vi "Main.vi"() -> ()   [LabVIEW 2024]
uses:
  SubVIs/Typdefinitionen/Zustand.ctl
  SubVIs/Typdefinitionen/Registerkartenelement.ctl
  SubVIs/Typdefinitionen/Cluster_SPS_IN.ctl
  SubVIs/Typdefinitionen/Befehl_Lichtgitter.ctl
  SubVIs/Typdefinitionen/Cluster_out_Lichtgitter.ctl
  SubVIs/Typdefinitionen/Statistik.ctl
  SubVIs/Typdefinitionen/Cluster_SPS_OUT.ctl
  <vilib>/vision/Image Controls.llb/IMAQ Image.ctl
  SubVIs/Sonstige/Globale Variablen.vi
  <vilib>/vision/driver/NI_Vision_Acquisition_Software.lvlib
panel:
  out "error out":errorcluster
  in  "Registerkarte":T1
  in  "Start Kamera Unten":bool
  in  "Start Position":bool
  in  "Start Lichtgitter":bool
  in  "Zoom zurücksetzen":bool
  in  "Registerkarte Bilder":enum32{"Prüfungen", "Rohbilder"}(tab)
  out "Nachprüfung von Unten":T2(plugin-control)
  out "Ermittlung Kontaktposition":T2(plugin-control)
  out "Rohbild ISO":T2(plugin-control)
  out "Rohbild Referenzmarken":T2(plugin-control)
  out "Zeit Position ermitteln (ms)":u32
  out "Zeit Lichtgitter (ms)":u32
  out "Zeit Kamera Unten (ms)":u32
  in  "Größe Kontaktsuchfeld":sgl=70.0
  out "Artikelnummer & Fertigungsauftrag":T3={"Artikelnummer"="Test", "Fertigungsauftrag"="Test"}
  out "Messdaten":T4 {"Durchmesser Kontakt" format="%#.3f"; "Durchmesser Loch" format="%#.3f"; "Winkel Kontakt" format="%#.0f"; "Offset"."x" format="%#.3f"; "Offset"."y" format="%#.3g"; "Position Kontakt"."x" format="%#.3f"; "Position Kontakt"."y" format="%#.3f"}
  in  "Offline":T5={"Start Gesamtablauf"=FALSE, "Teile-Nummer"=0, "Teile-Datum"=0, "Kontaktnummer"=1} {"Kontaktnummer" min=1 max=40 step=1; "Teile-Datum" items=["09.12.24"]; "Teile-Nummer" max=0 step=1}
  out "Statistik Anlage":T6
  out "Statistik Artikel":T6
  out "Statistik Auftrag":T6
  out "SPS IN":T7
  out "SPS OUT":T8
  in  "Bildspeicherung Offline":bool
  in  "Cluster beobachten":bool
  in  "Lichtgitter manuell ansteuern":bool
  in  "Befehl:":T9
  out "Ergebnisse:":T10
  in  "ID Messverstärker":u32=1 min=1 max=2
  in  "Artikelnummer Offline":string="Test"
  in  "i. O. Bilder speichern":bool
  in  "SubVI öffnen":bool
  in  "Livebild":bool
  out "Zustand":T11=enum."Bild Unten speichern"
  out "Programmversion":string
  in  "ACK":bool
  out "Beschreibung:":string
  in  "Fehlercode:":string
  out "Fehler Beenden":errorcluster
  in  "Flüssiglinse neu verbinden":bool
  out "Fehler Flüssiglinse":errorcluster
  in  "Lichtgitter neu verbinden":bool
  in  "SPS neu verbinden":bool
  in  "Kamera Oben neu verbinden":bool
  in  "Kamera Unten neu verbinden":bool
  out "Fehler Lichtgitter":errorcluster
  out "Fehler SPS":errorcluster
  out "Fehler Kamera Unten":errorcluster
  out "Fehler Kamera Oben":errorcluster
  out "Fehler init allgemein":errorcluster
  out "Fehler Nebenschleife":errorcluster
  out "Fehler Main":errorcluster
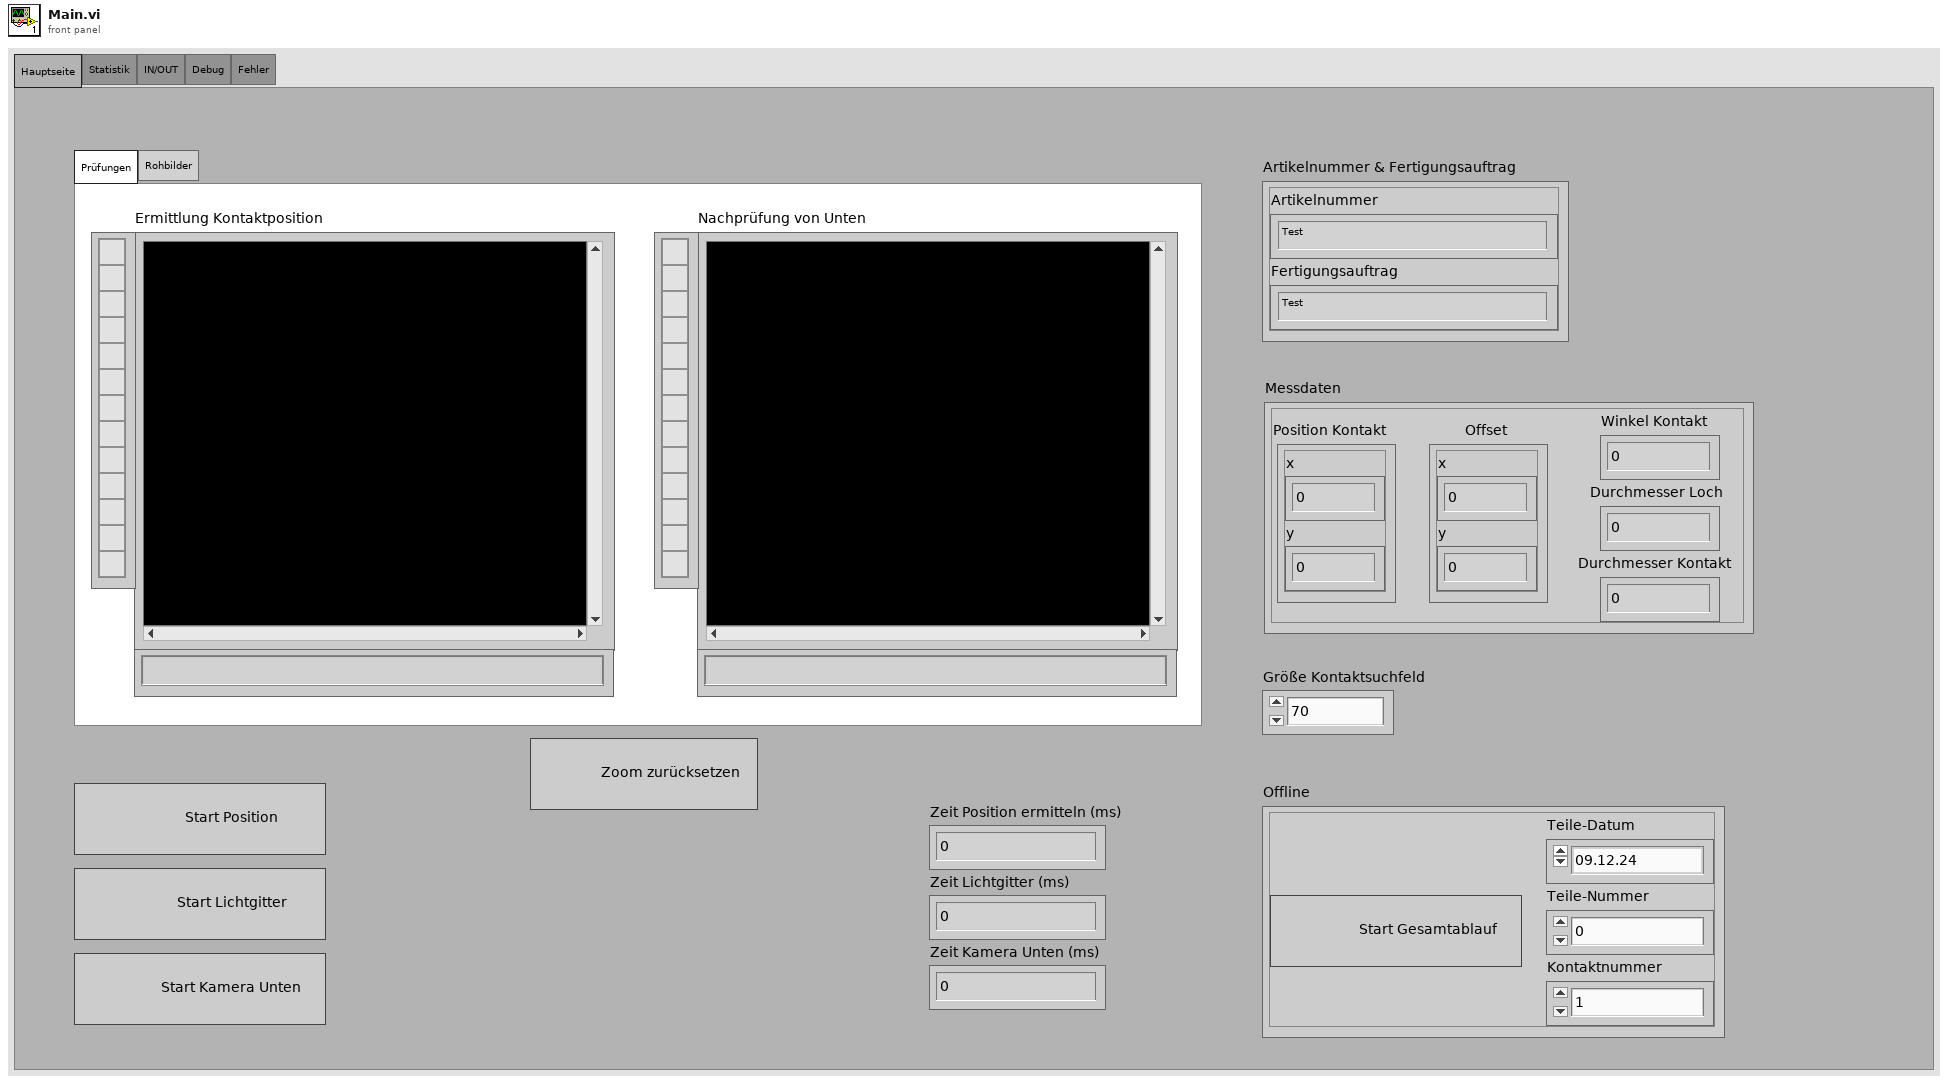
[diagram p1: front panel]
types:
  T1 = typedef "Registerkartenelement.ctl" = enum32{"Hauptseite", "Statistik", "IN/OUT", "Debug", "Fehler"}
  T2 = typedef "IMAQ Image.ctl" = refnum<image>
  T3 = cluster{"Artikelnummer":string, "Fertigungsauftrag":string}
  T4 = cluster{"Position Kontakt":cluster{"x":dbl, "y":dbl}, "Offset":cluster{"x":dbl, "y":dbl}, "Winkel Kontakt":dbl, "Durchmesser Loch":dbl, "Durchmesser Kontakt":dbl}
  T5 = cluster{"Start Gesamtablauf":bool, "Teile-Nummer":u32, "Teile-Datum":u16, "Kontaktnummer":u32}
  T6 = typedef "Statistik.ctl" = cluster{"Bestückte ISO":u32, "Verbaute Kontakte":u32, "ISO n.i.O.":u32, "Nachkontrolle Unten n.i.O":u32, "Position nicht gefunden":u32}
  T7 = typedef "Cluster_SPS_IN.ctl" = cluster{"Artikelnummer":string, "Fertigungsauftrag":string, "Start Position ermitteln":bool, "Start Kontaktvermessung Lichtgitter":bool, "Start Nachkontrolle":bool, "ACK SPS":bool}
  T8 = typedef "Cluster_SPS_OUT.ctl" = cluster{"Koordinaten ermittelt":bool, "Nachkontrolle Kamera Unten fertig":bool, "Vermessung Lichtgitter fertig":bool, "Position x":dbl, "Position y":dbl, "Winkel Kontakt":dbl, "Offset x":dbl, "Offset y":dbl, "Referenzen nicht gefunden":bool, "Kontaktposition nicht gefunden":bool, "Kontakt nicht in Lichtgitter":bool, "Kontakt zu klein":bool, "Kontakt zu groß":bool, "Kamera Unten n.i.O.":bool}
  T9 = typedef "Befehl_Lichtgitter.ctl" = enum16{"Anzahl Messverstärker ermitteln", "Aktuellen Messwert von einem Messverstärker lesen", "Aktuellen Messwerte von allen Messverstärkern lesen", "Anzahl Kanten von einem Messverstärker ermitteln", "Alle Kanten von allen Messverstärkern lesen"}
  T10 = typedef "Cluster_out_Lichtgitter.ctl" = cluster{"Anzahl Messverstärker":i32, "Messwert in mm":dbl, "Alle Messwerte in mm":dbl[], "Anzahl Kanten":i32, "Messwerte out":dbl[][]}
  T11 = typedef "Zustand.ctl" = enum16{"Warten auf Event", "Artikeldaten laden", "Init Prüfung Oben", "Bildaufnahme Oben", "Auswertung Oben", "Bilder Oben speichern", "Init Vermessung Lichtgitter", "Messwertaufnahme Lichtgitter", "Auswertung Lichtgitter", "Init Prüfung Unten", "Bildaufnahme Unten", "Auswertung Unten", "Bild Unten speichern", "Update Statistik", "Fehler quittieren"}
  T12 = enum32{"invalid app kind", "Development System", "Run Time System", "Student Edition", "Embedded LabVIEW", "Evaluation", "Custom"}
  T13 = typedef "Cluster_Fehler_Initialisierung.ctl" = cluster{"Fehler init allgemein":errorcluster, "Fehler Kamera Oben init":errorcluster, "Fehler Flüssiglinse init":errorcluster, "Fehler Kamera Unten init":errorcluster, "Fehler SPS init":errorcluster, "Fehler Lichtgitter init":errorcluster}
  T14 = typedef "Cluster.ctl" = cluster{"Initialisierung":cluster{"Online?":bool, "Grundpfad":path, "Kamera Oben":T15, "IP-Adresse Flüssiglinse":string, "Flüssiglinse":refnum<k5>, "Kamera Unten":T15, "IP-Adresse SPS":string, "SPS-Verbindung":T16, "IP-Adresse Lichtgitter":string, "Lichtgitter":refnum<k5>, "Skalierungsfaktor":dbl, "Bilder Oben":T2[], "Bild Unten":T2, "Bild Ausschnitt Unten":T2}, "Einstellungen":cluster{"Gesamtablauf gestartet":bool, "i. O. Bilder speichern":bool, "Bildspeicherung Offline":bool, "Ausgewähltes Offline-Datum":string, "Ausgewähltes Offline-Teil":string, "Speicherpfad Bilder":path}, "Artikeldaten":cluster{"Artikelnummer":string, "Fertigungsauftrag":string, "Muster ISO":T2, "Belichtungszeit Referenzmarken":dbl, "Fokus Referenzmarken":dbl, "Belichtungszeit ISO":dbl, "Fokus ISO":dbl, "Belichtungszeit Unten":dbl, "Kontaktanzahl":u32, "Aktueller Kontakt":i16, "Kontaktposition":cluster{"x":sgl, "y":sgl}, "ISO-Muster nicht vorhanden":bool, "Winkel ISO":sgl, "Mittelpunkt ISO":cluster{"x":dbl, "y":dbl}}, "Werte Kamera Oben":cluster{"Koordinatensystem":T19, "Position Kontakt":cluster{"x":dbl, "y":dbl}, "Durchmesser Loch":dbl, "Winkel Kontakt":dbl, "Position Kontakt umgerechnet":cluster{"x":dbl, "y":dbl}}, "Werte Kamera Unten":cluster{"Prüfung Unten n. i. O.":bool}, "Werte Lichtgitter":cluster{"Messwerte Referenzmarken":dbl[][], "Mittelpunkt Referenzmarken":cluster{"x":dbl, "y":dbl}, "Messwerte Kontakt":dbl[][], "Offset":cluster{"x":dbl, "y":dbl}}, "Rückmeldungen":cluster{"Koordinaten ermittelt":bool, "Vermessung Lichtgitter fertig":bool, "Nachkontrolle Kamera Unten fertig":bool}, "Fehler":cluster{"Referenzen nicht gefunden":bool, "Kontakt nicht gefunden":bool, "Referenzen nicht in Lichtgitter":bool, "Kontakt zu groß":bool, "Kontakt zu klein":bool}, "Statistik":cluster{"Statistiken":T6[]}, "Timer":cluster{"Timer Start Position":u32, "Timer Start Lichtgitter":u32, "Timer Start Kamera Unten":u32}}
  T15 = typedef "IMAQdx.ctl" = refnum<k21>
  T16 = typedef "SP7.lvlib/S7 Connection.ctl" = cluster{"TCP Connection Ref":refnum<k5>, "IP address":string, "timeout ms":i32, "Connected?":bool, "PLC Type":T17, "Rack S7 400":u8, "Slot S7 400":u8, "PDU Size":u16, "connection semaphore":T18}
  T17 = typedef "SP7.lvlib/PLC Type.ctl" = enum16{"S7 200", "S7 300/400", "S7 1200", "S7 1500", "LOGO!8"}
  T18 = typedef "Semaphore RefNum" = refnum<k1>
  T19 = typedef "Koordinatensystem.ctl" = cluster{"Punkt x-Achse":cluster{"X":sgl, "Y":sgl}, "Ursprung":cluster{"X":sgl, "Y":sgl}, "Punkt y-Achse":cluster{"X":sgl, "Y":sgl}}
  T20 = cluster{"Referenzen nicht gefunden":bool, "Kontakt nicht gefunden":bool, "Kontakt nicht in Lichtgitter":bool, "Kontakt zu groß":bool, "Kontakt zu klein":bool}
  T21 = cluster{"Messwerte Referenzmarken":dbl[][], "Mittelpunkt Referenzmarken":cluster{"x":dbl, "y":dbl}, "Messwerte Kontakt":dbl[][], "Offset":cluster{"x":dbl, "y":dbl}}
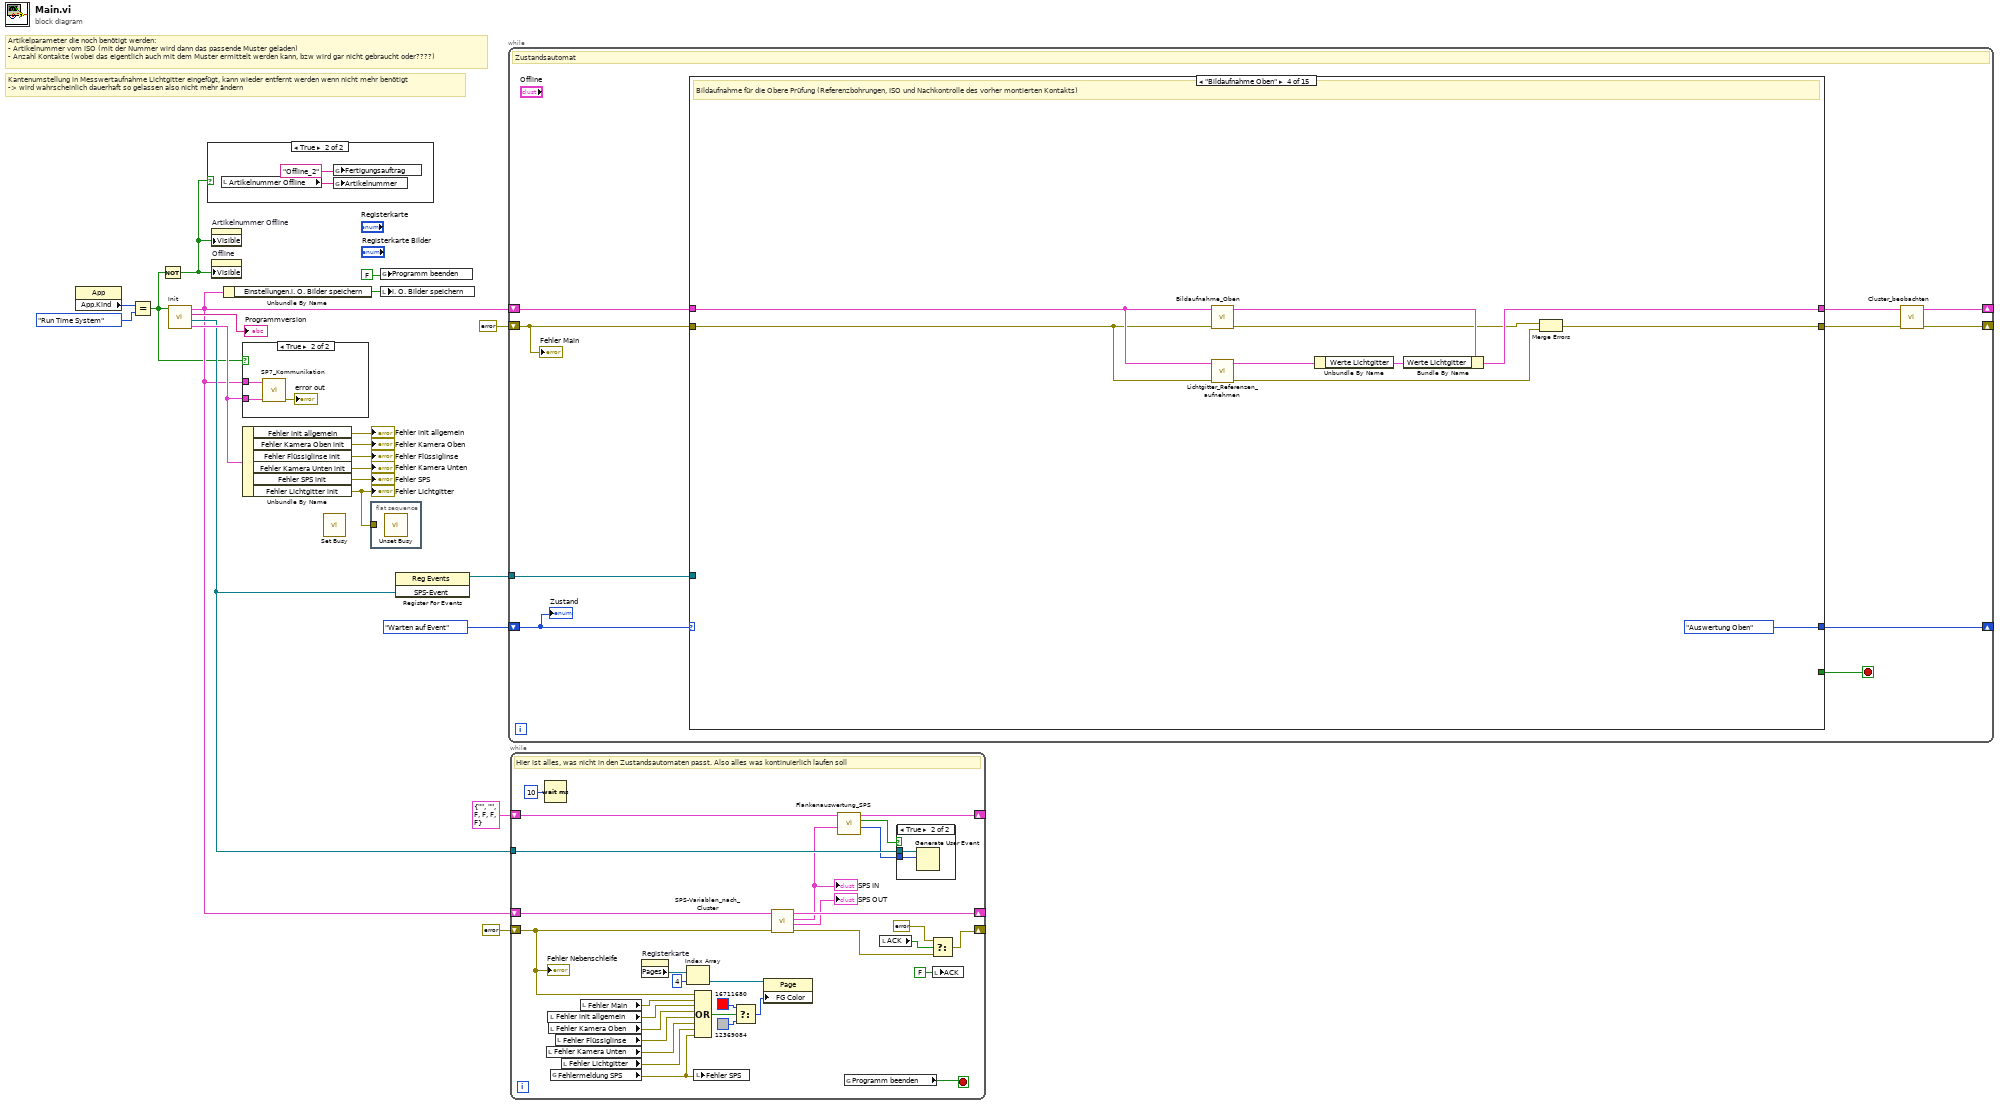
[diagram p0: block diagram]
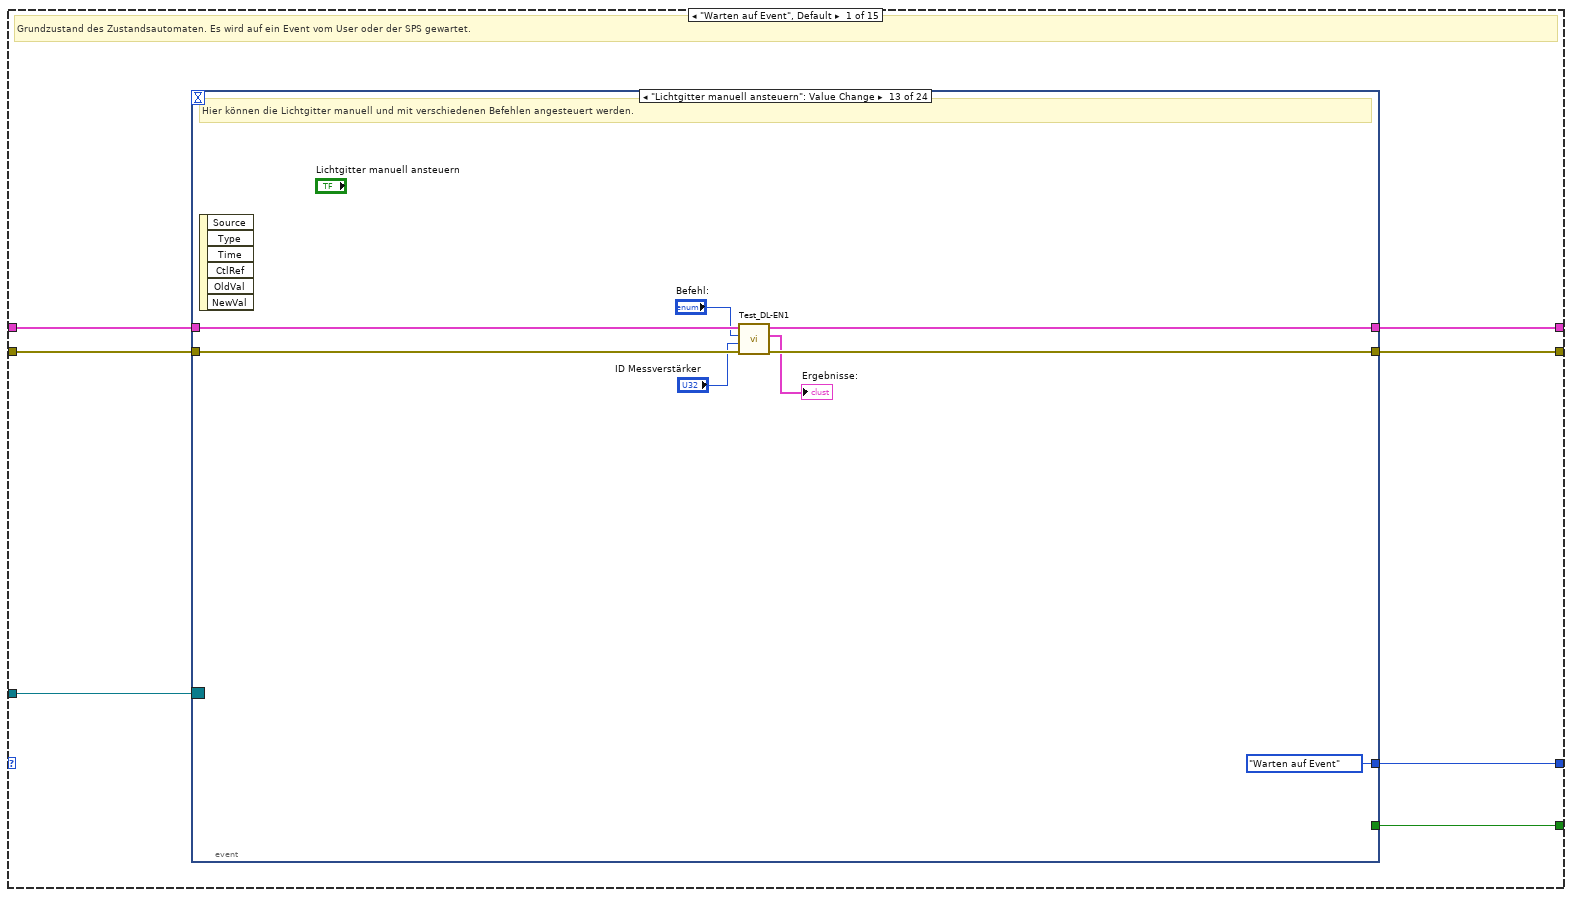
[diagram p2: hidden frame]
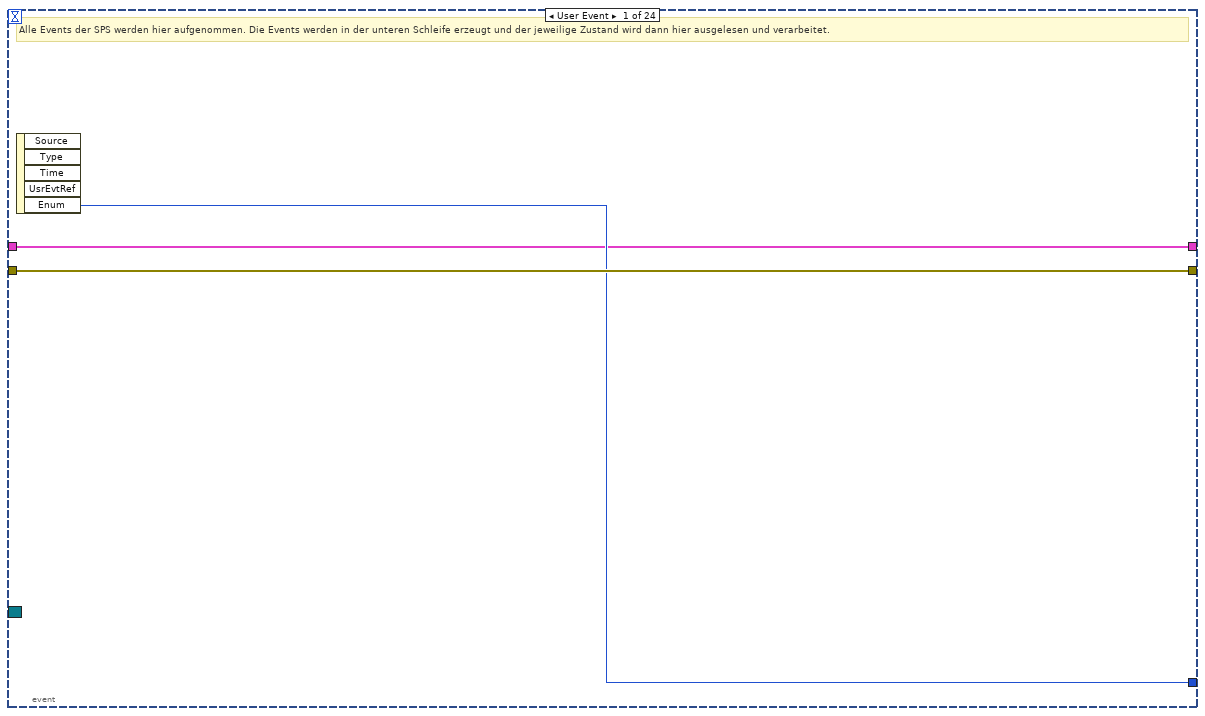
[diagram p3: hidden frame]
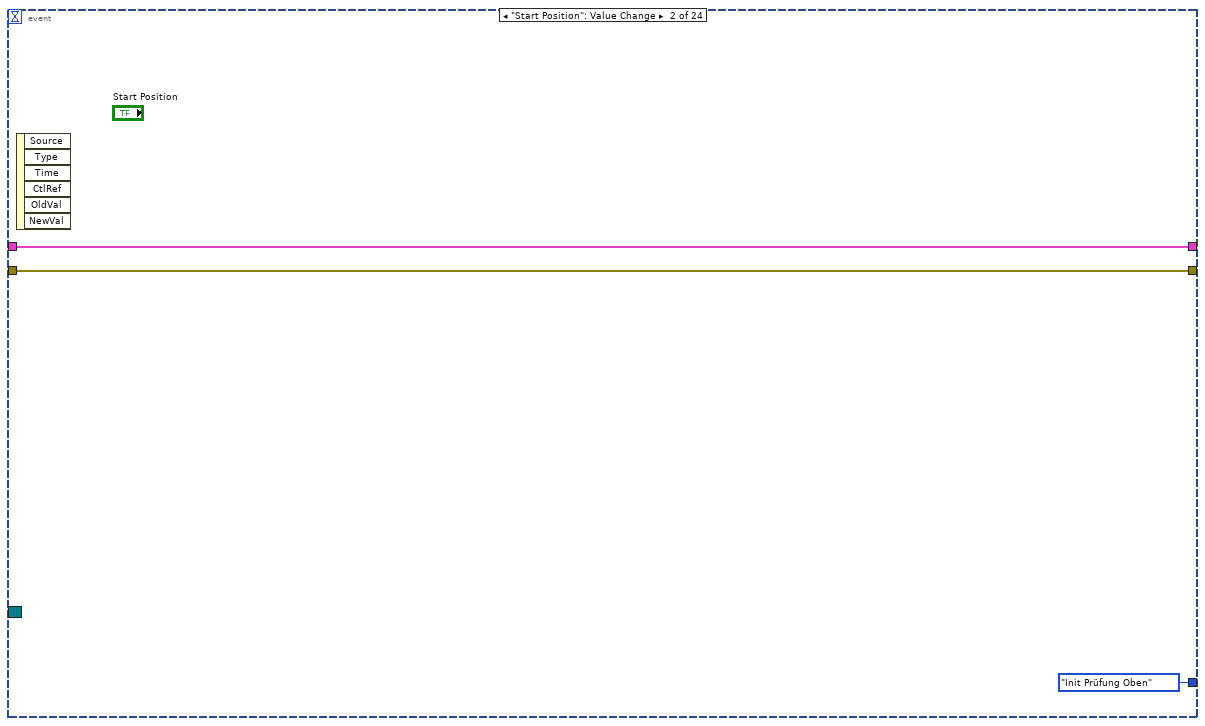
[diagram p4: hidden frame]
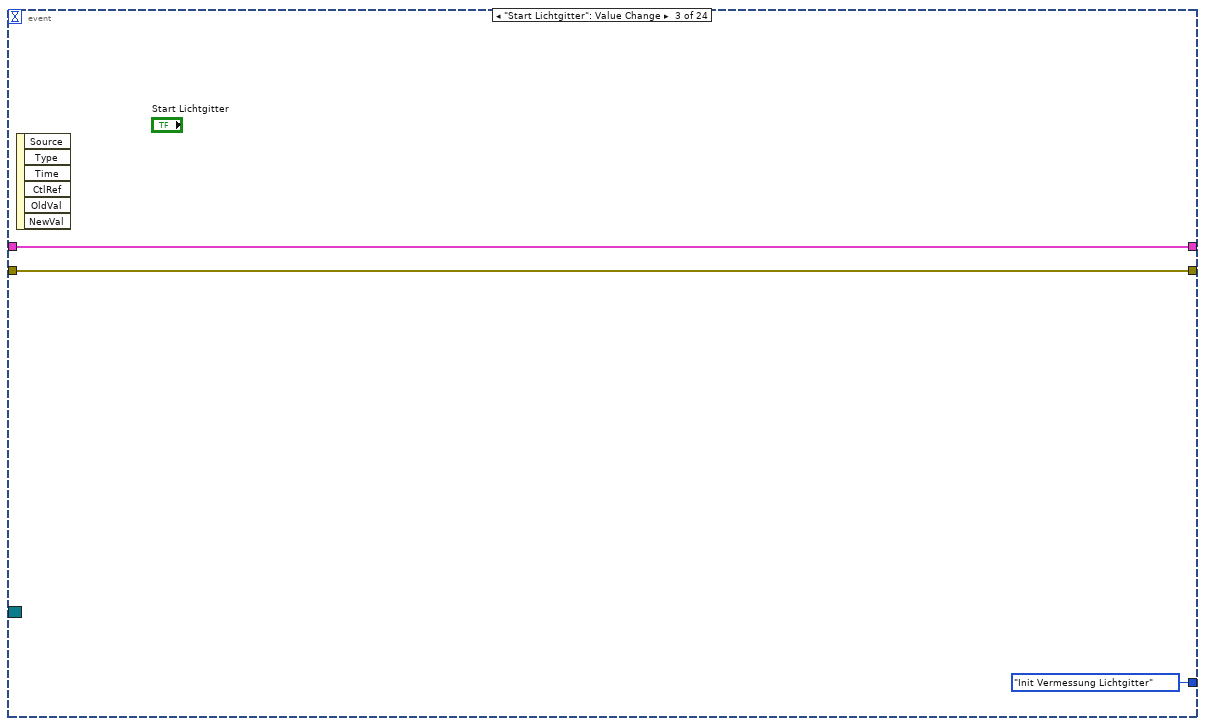
[diagram p5: hidden frame]
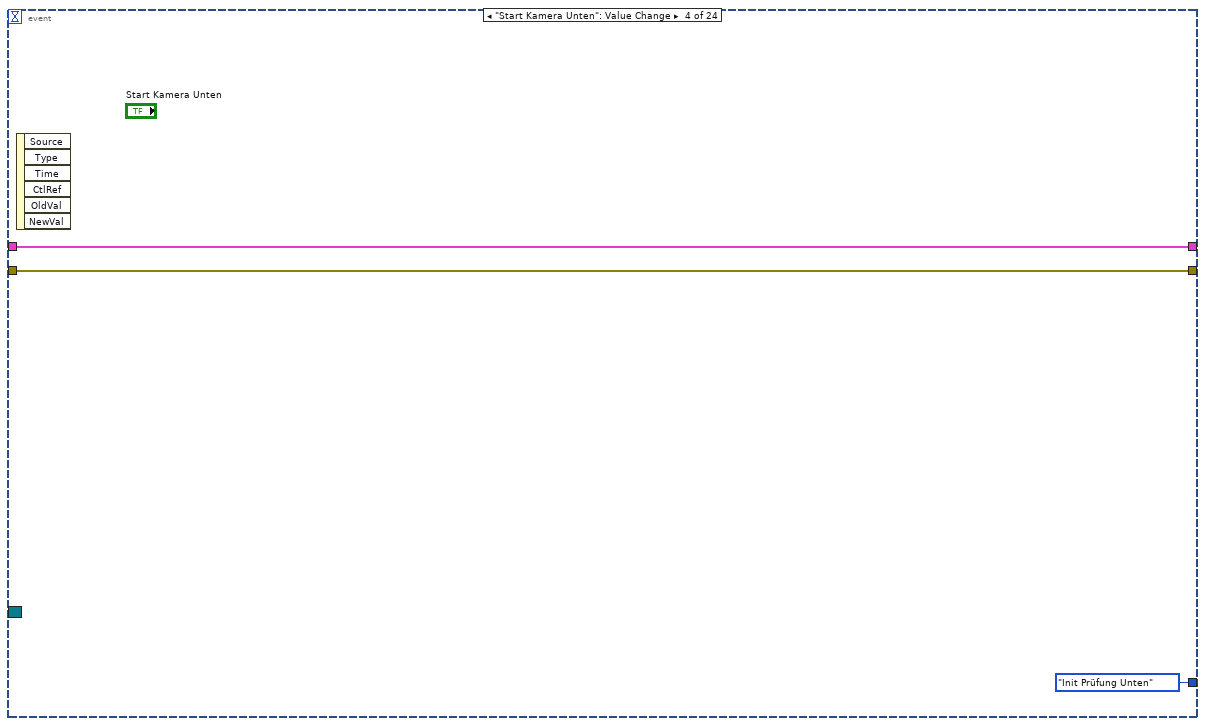
[diagram p6: hidden frame]
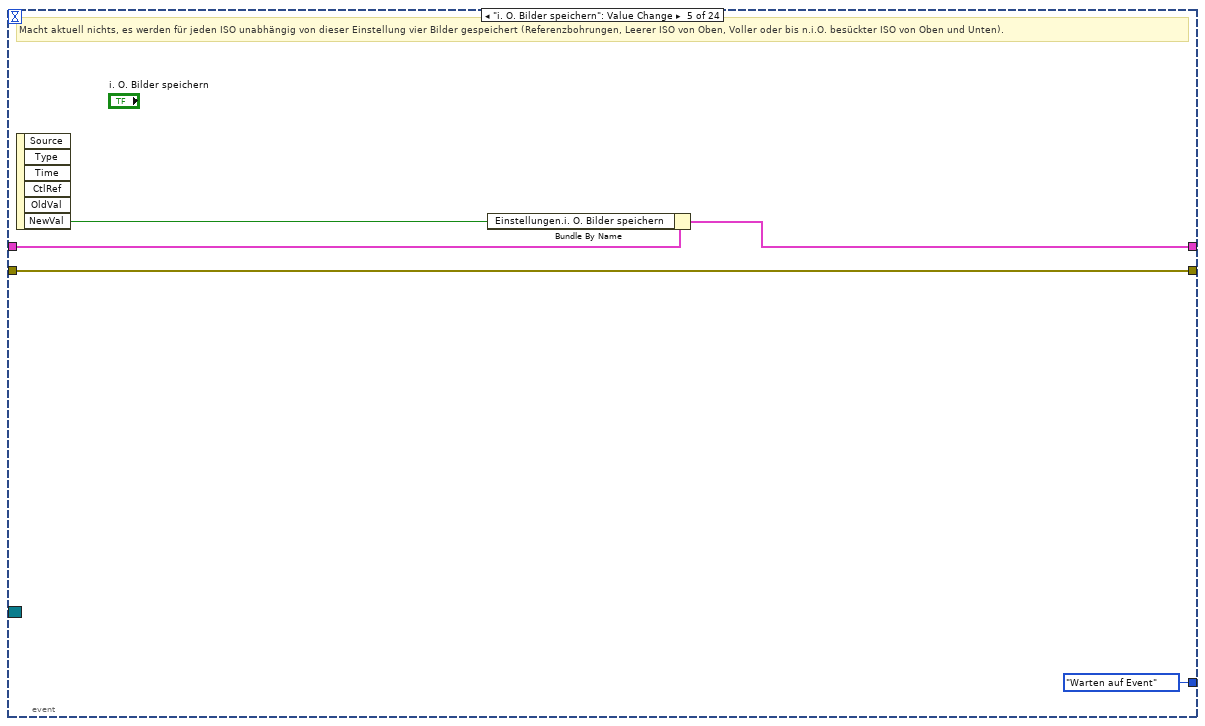
[diagram p7: hidden frame]
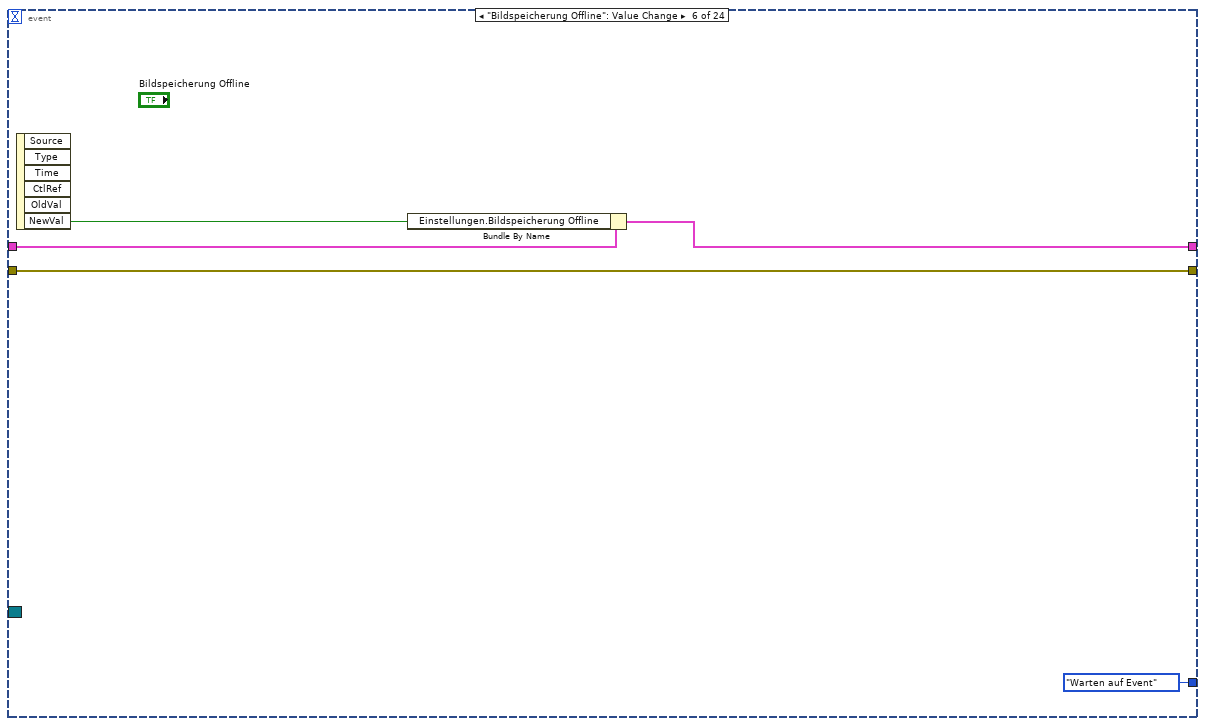
[diagram p8: hidden frame]
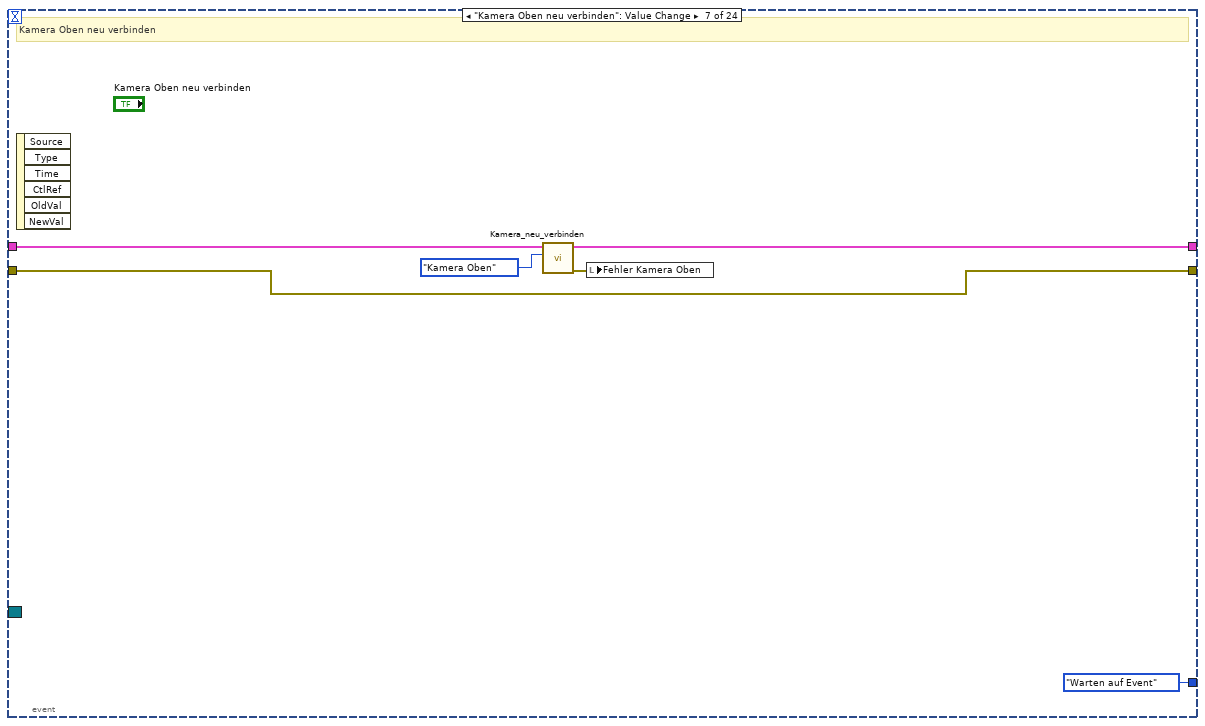
[diagram p9: hidden frame]
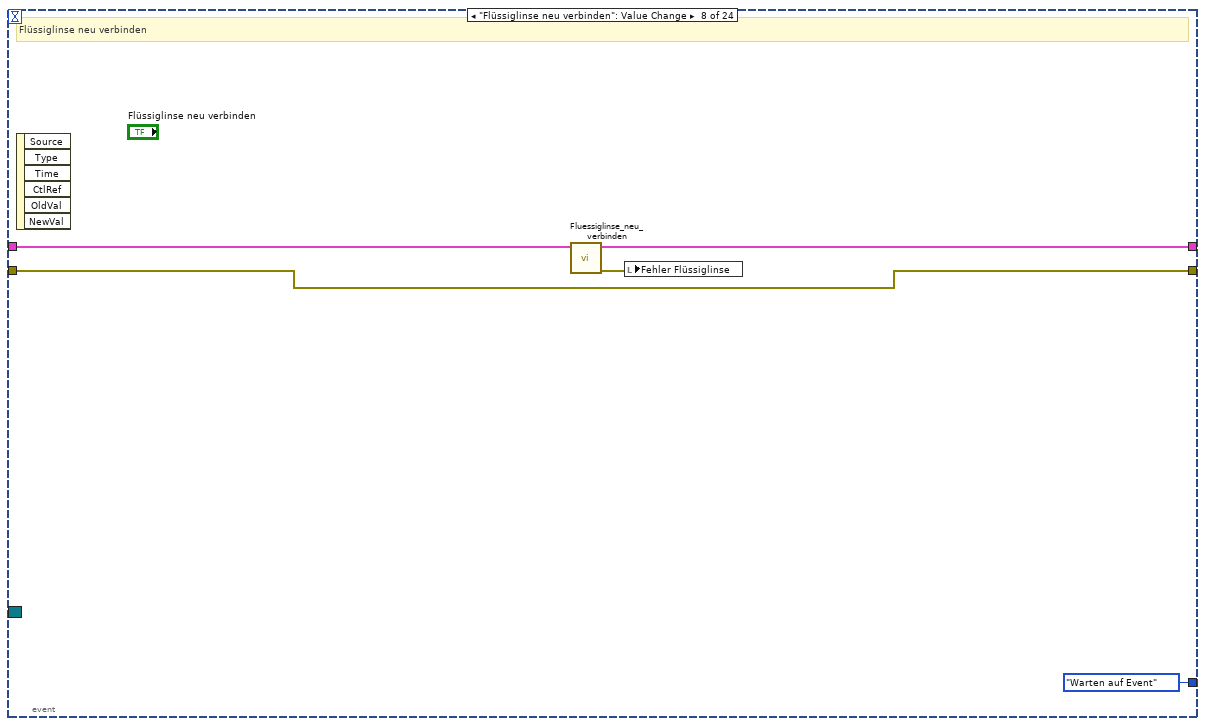
[diagram p10: hidden frame]
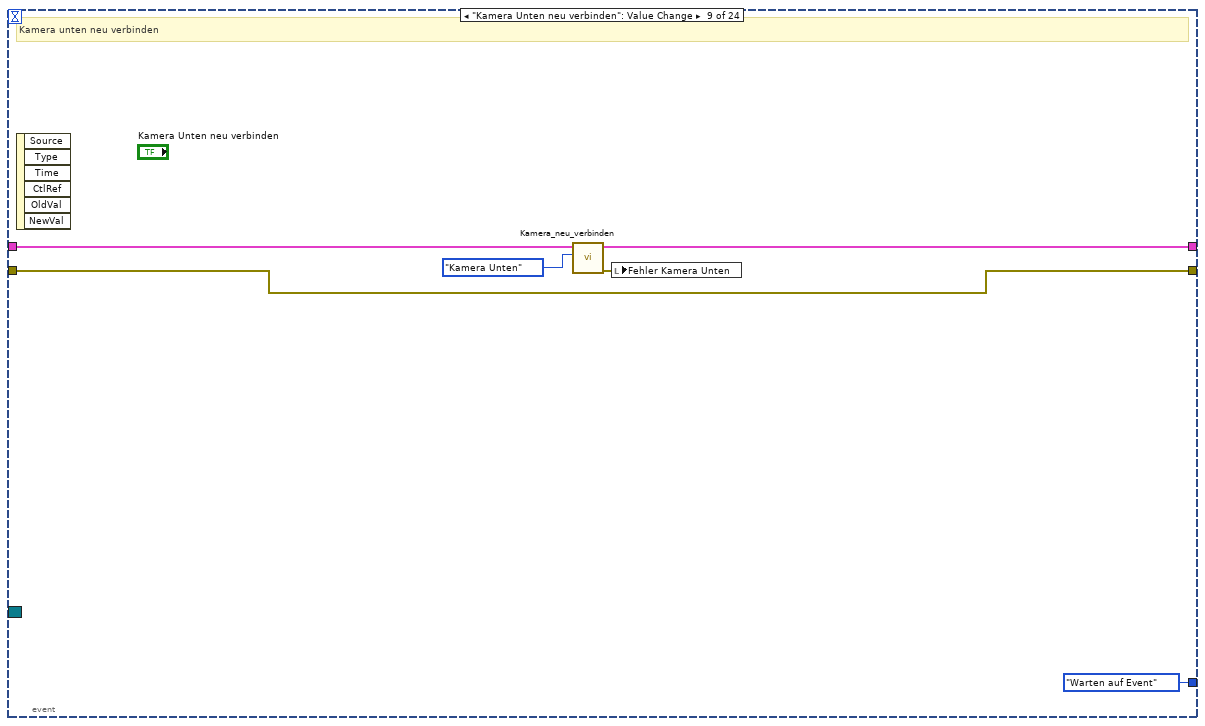
[diagram p11: hidden frame]
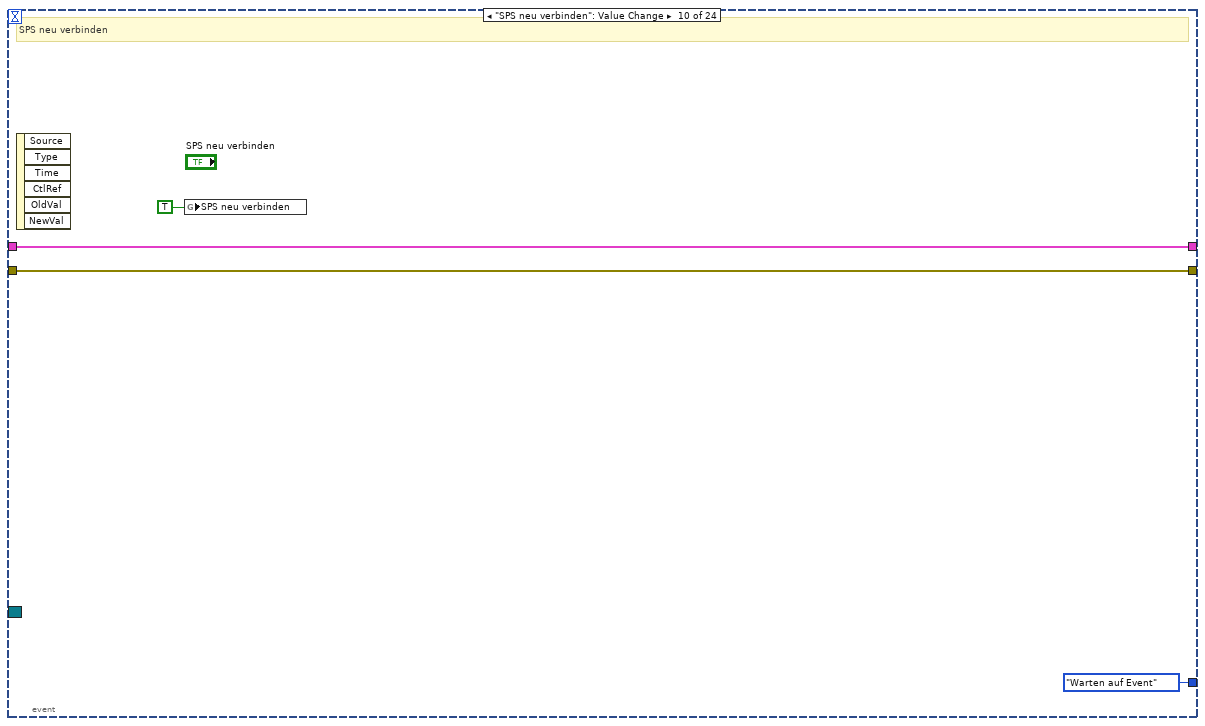
[diagram p12: hidden frame]
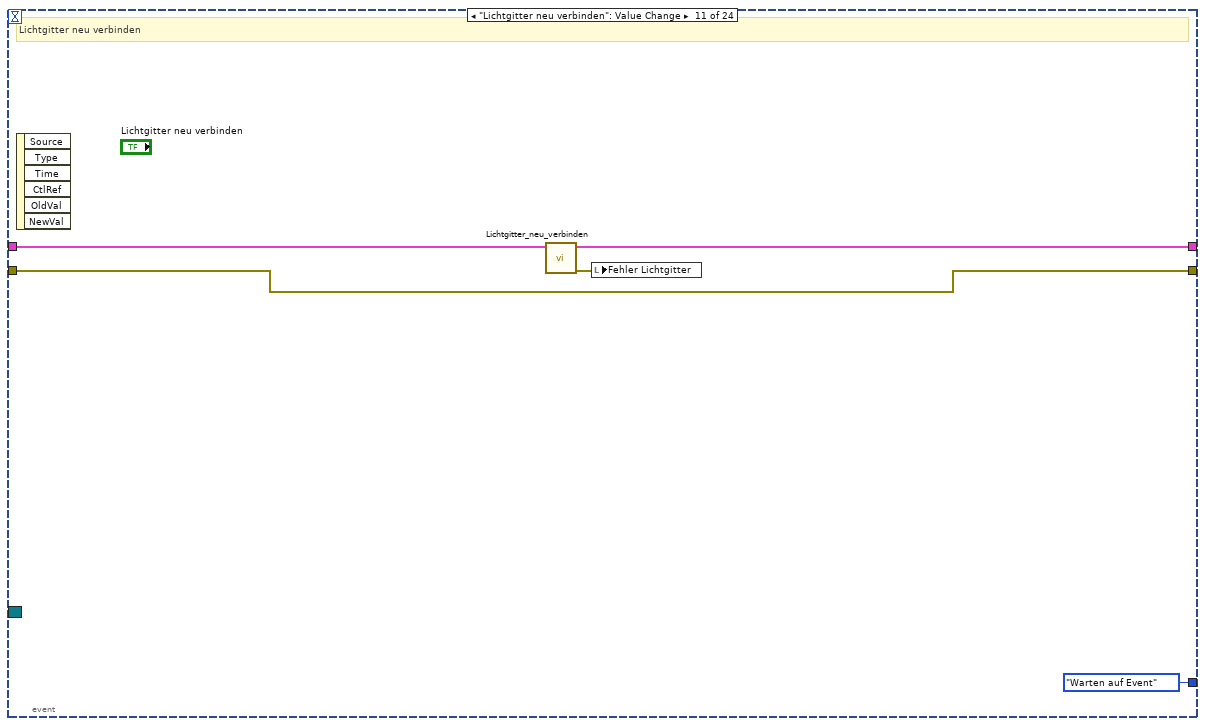
[diagram p13: hidden frame]
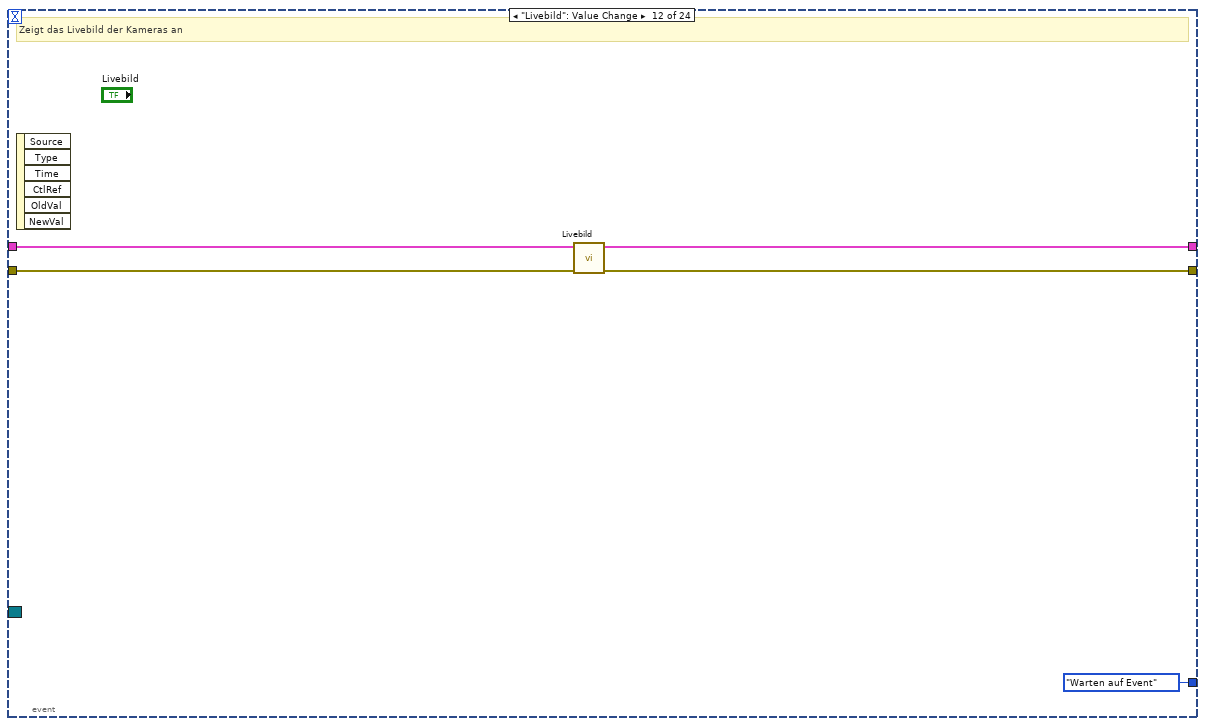
[diagram p14: hidden frame]
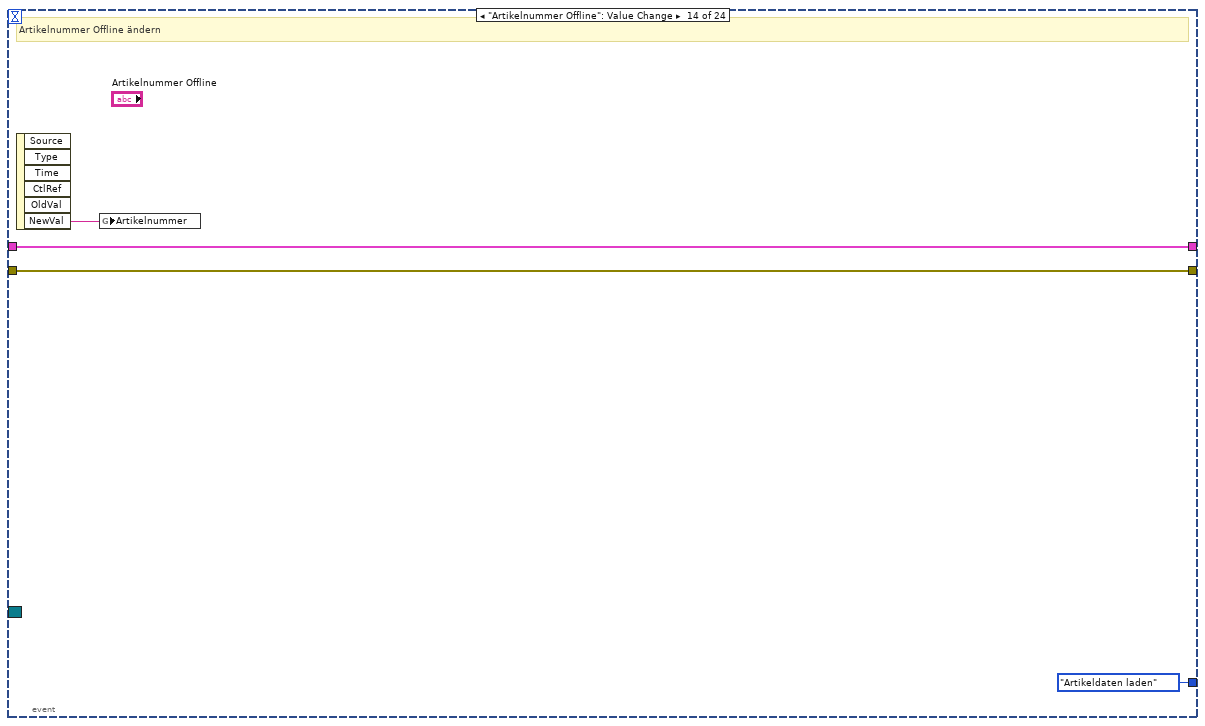
[diagram p15: hidden frame]
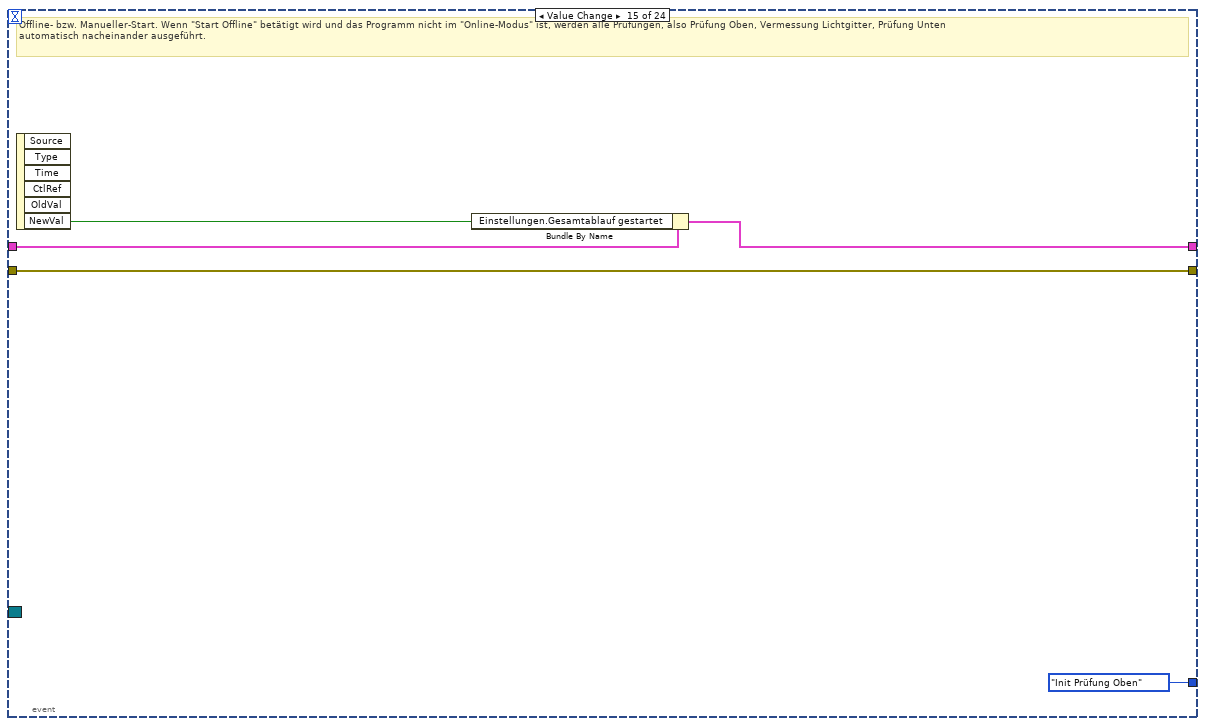
[diagram p16: hidden frame]
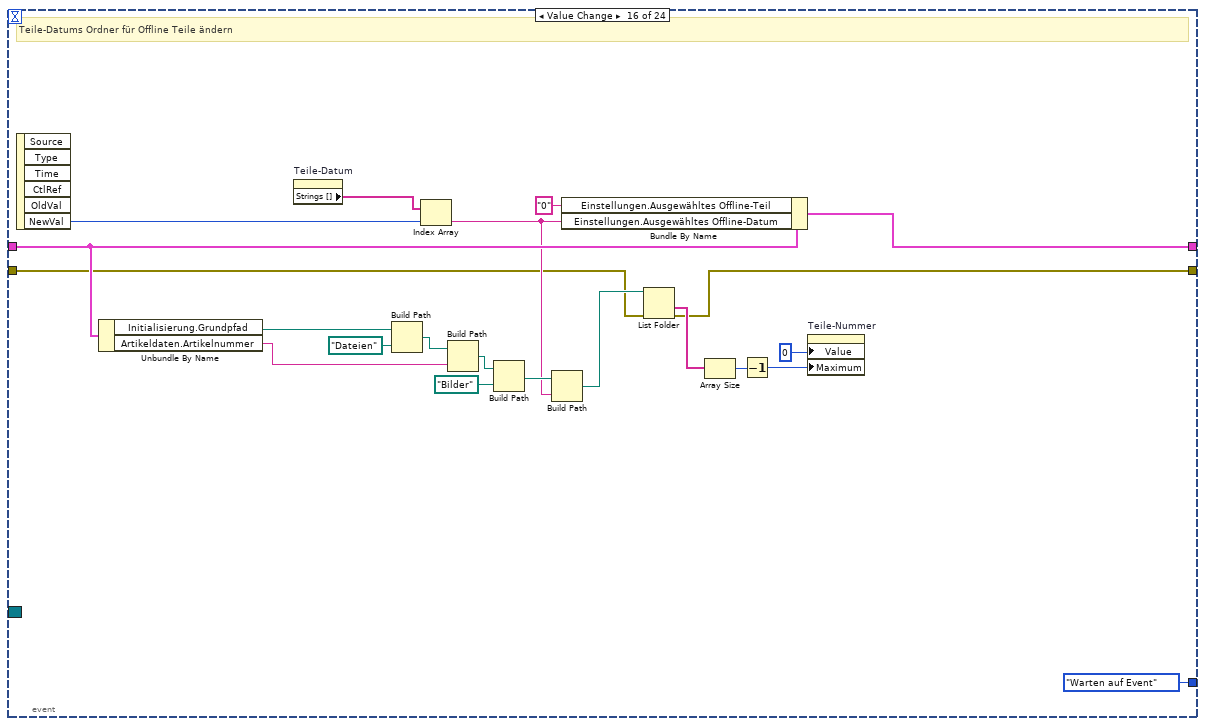
[diagram p17: hidden frame]
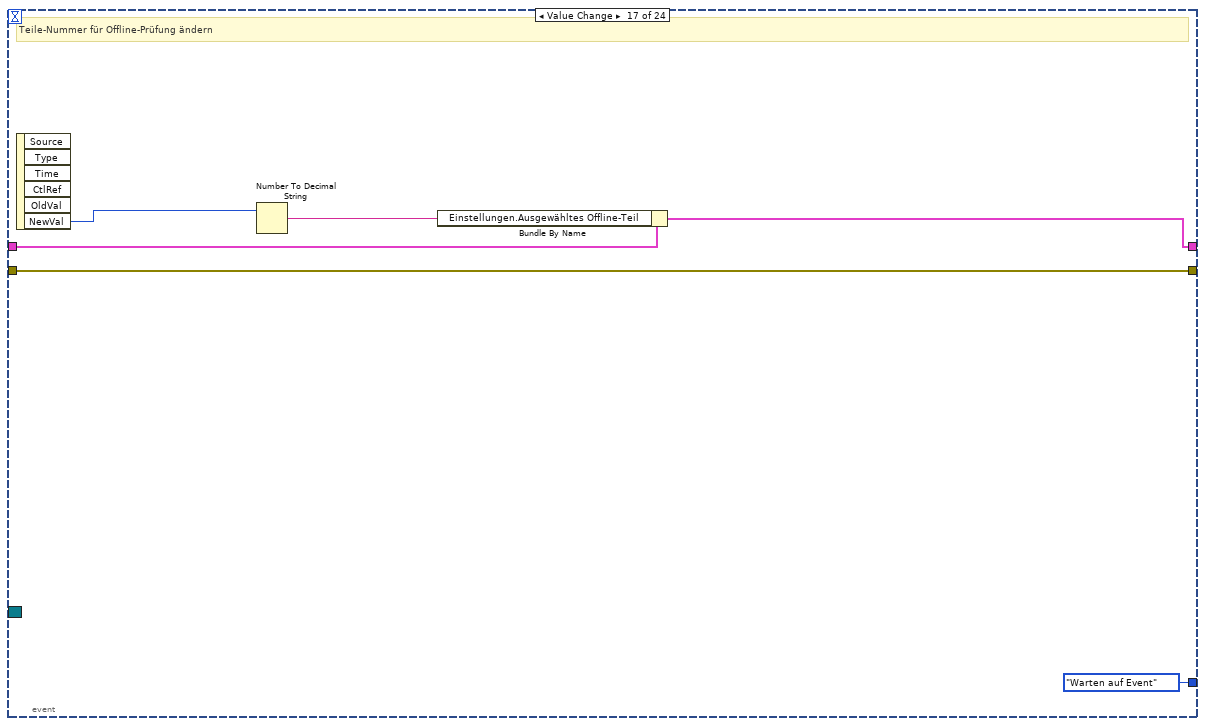
[diagram p18: hidden frame]
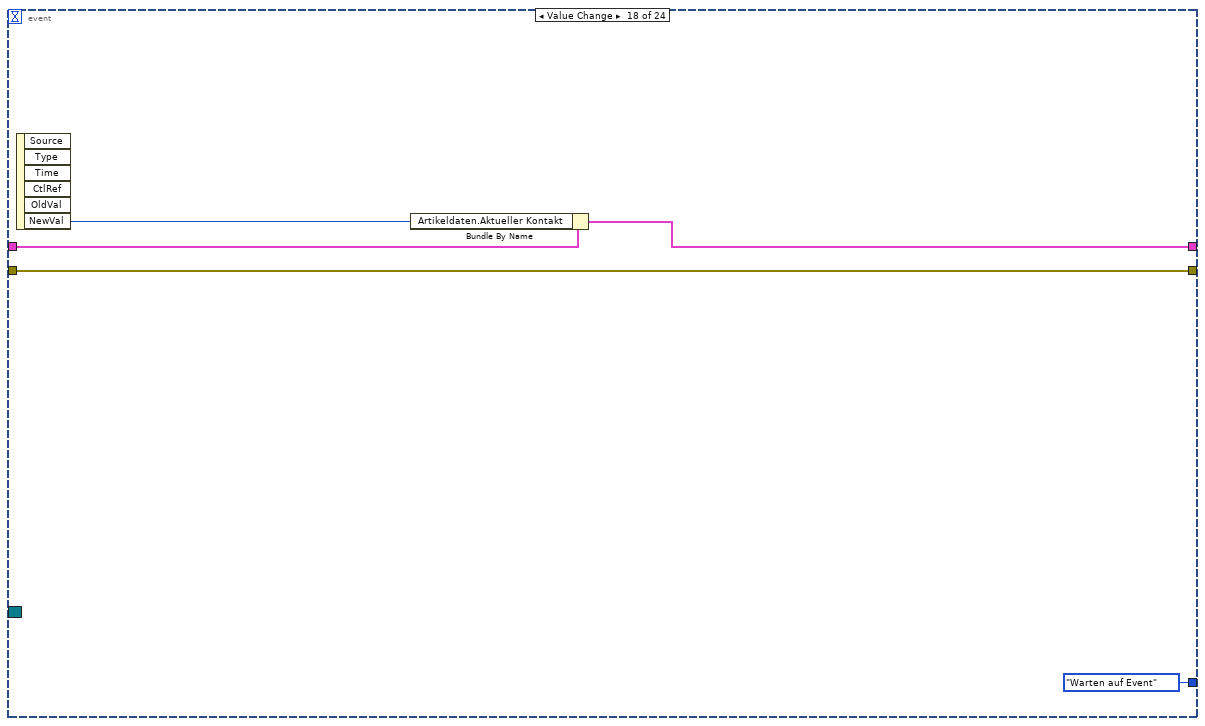
[diagram p19: hidden frame]
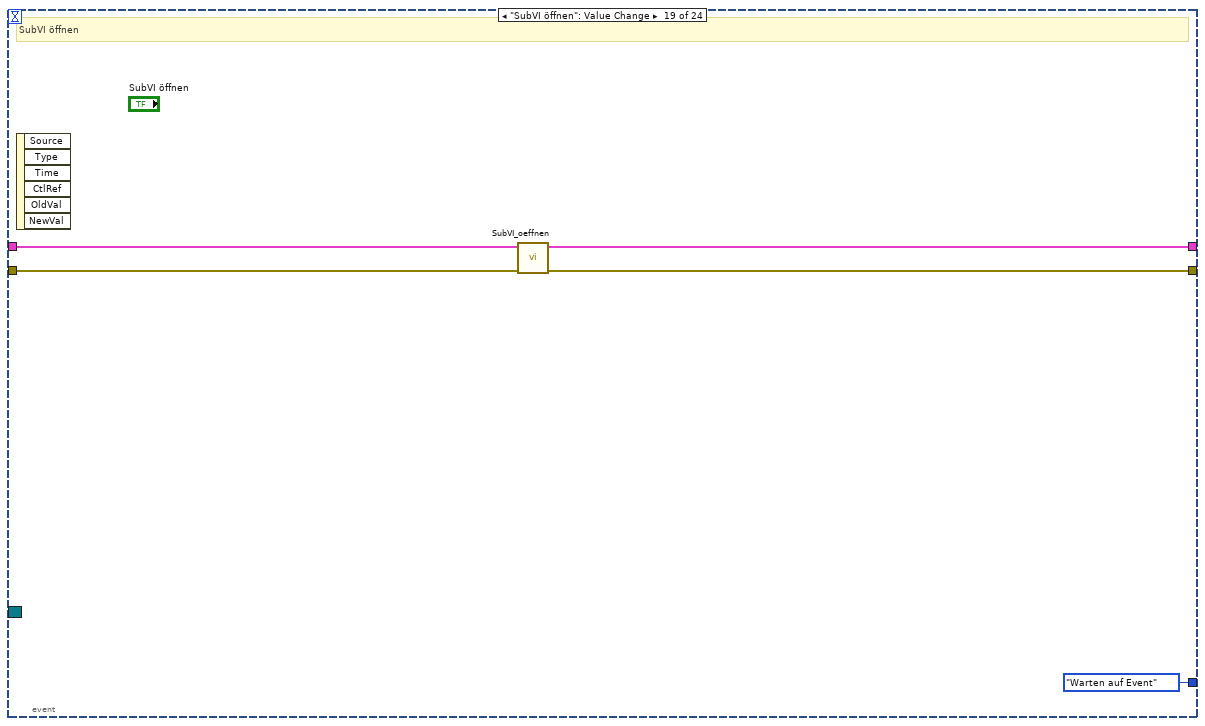
[diagram p20: hidden frame]
diagram:
  # "Kantenumstellung in Messwertaufnahme Lichtgitter eingefügt, kann wieder entfernt werden wenn nicht mehr benötigt\n-> wird wahrscheinlich dauerhaft so gelassen also nicht mehr ändern"
  # "Artikelparameter die noch benötigt werden:\n- Artikelnummer vom ISO (mit der Nummer wird dann das passende Muster geladen)\n- Anzahl Kontakte (wobei das eigentlich auch mit dem Muster ermittelt werden kann, bzw wird gar nicht gebraucht oder????)"
  n1 = property class="App"() -> ("App.Kind"=w13:T12)  [unwired: 2 in, 2 out]
  n2 = Equal?(x=w13, y=T12."Run Time System") -> (x = y?=w4:bool)
  n3 = Not(x=w4) -> (.not. x?=w1:bool)
  n4 = call "Init.vi"("Online?"=w4) -> ("Fehler out"=w17:T13, "SPS-Event"=w9:refnum<user-event>, "Version"=→"Programmversion":string, "Cluster out"=w6:T14)  [unwired: 7 in]
  n5 = case shown="True" w1 {
    frame False {
    }
    frame True {
      n6 = local read "Artikelnummer Offline"() -> (w23:string)
      n7 = global write "Globale Variablen.vi" "Fertigungsauftrag"("Offline_2" ("Fertigungsauftrag")) -> ()
      n8 = global write "Globale Variablen.vi" "Artikelnummer"(w23) -> ()
    }
  }
  n9 = property on="Artikelnummer Offline" class="Str"("Visible"=w1) -> ()  [unwired: 2 in, 2 out]
  n10 = property on="Offline" class="Clust"("Visible"=w1) -> ()  [unwired: 2 in, 2 out]
  n11 = Unbundle By Name(w6) -> ("Einstellungen.i. O. Bilder speichern"=w7:bool)
  n12 = Unbundle By Name(w17) -> ("Fehler init allgemein"=→"Fehler init allgemein":errorcluster, "Fehler Kamera Oben init"=→"Fehler Kamera Oben":errorcluster, "Fehler Flüssiglinse init"=→"Fehler Flüssiglinse":errorcluster, "Fehler Kamera Unten init"=→"Fehler Kamera Unten":errorcluster, "Fehler SPS init"=→"Fehler SPS":errorcluster, "Fehler Lichtgitter init"=w3:errorcluster)
  "Fehler Lichtgitter" <- w3
  n13 = case shown="True" w4 {
    tunnel: w17 -> [_ w26]
    tunnel: w6 -> [_ w25]
    frame False {
    }
    frame True {
      n14 = call "SP7_Kommunikation.vi"("Fehler in"=w26, "Cluster in"=w25) -> ("error out"=→"error out":errorcluster)  [unwired: 9 in]
    }
  }
  n15 = call <vilib>:"Set Busy.vi"() -> ()  [unwired: 10 in, 2 out]
  n16 = flat-sequence {
    tunnel: w3 -> [_]
    frame #0 {
      n17 = call <vilib>:"Unset Busy.vi"() -> ()  [unwired: 11 in, 1 out]
    }
  }
  n18 = global write "Globale Variablen.vi" "Programm beenden"(FALSE ("Programm beenden")) -> ()
  n19 = local write "i. O. Bilder speichern"(w7) -> ()
  n20 = register-events(w9) -> (reference out=w10:refnum<event-registration>)  [unwired: 2 in, 1 out]
  n21 = while {
    shift-right: [w31] -> _
    shift-left: w6 -> [w33]
    shift-right: [w27] -> _
    shift-left: errorcluster {"status"=FALSE, "code"=0, "source"=""} ("error out") -> [w36]
    shift-right: [w30] -> _
    shift-left: Zustand."Warten auf Event" -> [w29]
    tunnel: w10 -> [w35]
    stop <- w32 stop-if-true
    # "Zustandsautomat"
    n22 = case shown="\"Bildaufnahme Oben\"" w29 {
      tunnel: [w43 Zustand."Warten auf Event" ("State") Zustand."Bildaufnahme Oben" ("State") Zustand."Auswertung Oben" ("State") w283 w294 Zustand."Messwertaufnahme Lichtgitter" ("State") Zustand."Auswertung Lichtgitter" ("State") w332 Zustand."Bildaufnahme Unten" ("State") w351 w372 Zustand."Update Statistik" ("State") Zustand."Warten auf Event" ("State") Zustand."Warten auf Event" ("State")] -> w30
      tunnel: w33 -> [w42 w231 w241 w251 w259 w303 w306 w315 w335 w345 w355 w371 w379 w389 w396]
      tunnel: w36 -> [w40 w229 w240 w250 w284 w302 w305 w314 w334 w341 w353 w370 w378 w391 _]
      tunnel: [w41 w221 w236 w247 w258 w299 w308 w313 w327 w343 w354 w358 w376 w388 w398] -> w34
      tunnel: [w39 w230 w237 w244 w260 w301 w309 w312 w322 w342 w352 w356 w377 w390 w397] -> w28
      tunnel: w35 -> [w38 _ _ _ _ _ _ _ _ _ _ _ _ _ _]
      tunnel: [w37 _ _ _ _ _ _ _ _ _ _ _ _ _ _] -> w32
      frame "Warten auf Event", Default {
        # "Grundzustand des Zustandsautomaten. Es wird auf ein Event vom User oder der SPS gewartet."
        n23 = event shown="[12] \"Lichtgitter manuell ansteuern\": Value Change" {
          selector: w38 -> [_ _ _ _ _ _ _ _ _ _ _ _ _ _ _ _ _ _ _ _ _ _ _ _]
          dyn-events: _ -> [_ _ _ _ _ _ _ _ _ _ _ _ _ _ _ _ _ _ _ _ _ _ _ _]
          timeout: _ -> [_ _ _ _ _ _ _ _ _ _ _ _ _ _ _ _ _ _ _ _ _ _ _ _]
          tunnel: [w45 Zustand."Init Prüfung Oben" ("State") Zustand."Init Vermessung Lichtgitter" ("State") Zustand."Init Prüfung Unten" ("State") Zustand."Warten auf Event" ("State") Zustand."Warten auf Event" ("State") Zustand."Warten auf Event" ("State") Zustand."Warten auf Event" ("State") Zustand."Warten auf Event" ("State") Zustand."Warten auf Event" ("State") Zustand."Warten auf Event" ("State") Zustand."Warten auf Event" ("State") Zustand."Warten auf Event" ("State") Zustand."Artikeldaten laden" ("State") Zustand."Init Prüfung Oben" ("State") Zustand."Warten auf Event" ("State") Zustand."Warten auf Event" ("State") Zustand."Warten auf Event" ("State") Zustand."Warten auf Event" ("State") Zustand."Warten auf Event" ("State") Zustand."Warten auf Event" ("State") Zustand."Warten auf Event" ("State") Zustand."Fehler quittieren" ("State") Zustand."Warten auf Event" ("State")] -> w43
          tunnel: w42 -> [w44 w49 w52 w55 w58 w64 w70 w75 w80 w86 w90 w96 w103 w108 w109 w128 w139 w145 w150 w156 w173 w178 w183 w189]
          tunnel: [w44 w49 w52 w55 w57 w63 w69 w74 w81 w86 w89 w94 w101 w108 w110 w129 w138 w142 w147 w156 w173 w180 w183 w190] -> w41
          tunnel: w40 -> [w46 w48 w51 w54 w60 w65 w66 w73 w77 w85 w87 w95 w104 w107 w113 w118 w140 w141 w149 w160 w172 w179 w181 w192]
          tunnel: [w46 w48 w51 w54 w60 w65 w66 w73 w77 w85 w87 w93 w102 w107 w113 w114 w140 w141 w148 w159 w172 w177 w181 w191] -> w39
          tunnel: [_ _ _ _ _ _ _ _ _ _ _ _ _ _ _ _ _ _ _ _ _ _ _ TRUE] -> w37
          event User Event {
            # "Alle Events der SPS werden hier aufgenommen. Die Events werden in der unteren Schleife erzeugt und der jeweilige Zustand wird dann hier ausgelesen und verarbeitet."
            n24 = event-data() -> ("Enum"=w45:T11)  [unwired: 1 in, 4 out]
          }
          event "Start Position": Value Change {
            n25 = event-data() -> ()  [unwired: 1 in, 6 out]
          }
          event "Start Lichtgitter": Value Change {
            n26 = event-data() -> ()  [unwired: 1 in, 6 out]
          }
          event "Start Kamera Unten": Value Change {
            n27 = event-data() -> ()  [unwired: 1 in, 6 out]
          }
          event "i. O. Bilder speichern": Value Change {
            # "Macht aktuell nichts, es werden für jeden ISO unabhängig von dieser Einstellung vier Bilder gespeichert (Referenzbohrungen, Leerer ISO von Oben, Voller oder bis n.i.O. besückter ISO von Oben und Unten)."
            n28 = event-data() -> ("NewVal"=w56:bool)  [unwired: 1 in, 5 out]
            n29 = Bundle By Name(cluster=w58, "Einstellungen.i. O. Bilder speichern"=w56) -> (w57:T14)
          }
          event "Bildspeicherung Offline": Value Change {
            n30 = event-data() -> ("NewVal"=w62:bool)  [unwired: 1 in, 5 out]
            n31 = Bundle By Name(cluster=w64, "Einstellungen.Bildspeicherung Offline"=w62) -> (w63:T14)
          }
          event "Kamera Oben neu verbinden": Value Change {
            # "Kamera Oben neu verbinden"
            n32 = event-data() -> ()  [unwired: 1 in, 6 out]
            n33 = call "Kamera_neu_verbinden.vi"("Kamera"=enum16{"Kamera Oben", "Kamera Unten"}."Kamera Oben", "Cluster in"=w70) -> ("Fehler Kamera out"=w67:errorcluster, "Cluster out"=w69:T14)  [unwired: 8 in]
            n34 = local write "Fehler Kamera Oben"(w67) -> ()
          }
          event "Flüssiglinse neu verbinden": Value Change {
            # "Flüssiglinse neu verbinden"
            n35 = event-data() -> ()  [unwired: 1 in, 6 out]
            n36 = call "Fluessiglinse_neu_verbinden.vi"("Cluster in"=w75) -> ("Fehler Flüssiglinse out"=w72:errorcluster, "Cluster out"=w74:T14)  [unwired: 9 in]
            n37 = local write "Fehler Flüssiglinse"(w72) -> ()
          }
          event "Kamera Unten neu verbinden": Value Change {
            # "Kamera unten neu verbinden"
            n38 = event-data() -> ()  [unwired: 1 in, 6 out]
            n39 = call "Kamera_neu_verbinden.vi"("Kamera"=enum16{"Kamera Oben", "Kamera Unten"}."Kamera Unten", "Cluster in"=w80) -> ("Fehler Kamera out"=w78:errorcluster, "Cluster out"=w81:T14)  [unwired: 8 in]
            n40 = local write "Fehler Kamera Unten"(w78) -> ()
          }
          event "SPS neu verbinden": Value Change {
            # "SPS neu verbinden"
            n41 = event-data() -> ()  [unwired: 1 in, 6 out]
            n42 = global write "Globale Variablen.vi" "SPS neu verbinden"(TRUE ("Programm beenden")) -> ()
          }
          event "Lichtgitter neu verbinden": Value Change {
            # "Lichtgitter neu verbinden"
            n43 = event-data() -> ()  [unwired: 1 in, 6 out]
            n44 = call "Lichtgitter_neu_verbinden.vi"("Cluster in"=w90) -> ("Fehler Lichtgitter"=w88:errorcluster, "Cluster out"=w89:T14)  [unwired: 9 in]
            n45 = local write "Fehler Lichtgitter"(w88) -> ()
          }
          event "Livebild": Value Change {
            # "Zeigt das Livebild der Kameras an"
            n46 = event-data() -> ()  [unwired: 1 in, 6 out]
            n47 = call "Livebild.vi"("Fehler in"=w95, "Cluster in"=w96) -> ("Fehler out"=w93:errorcluster, "Cluster out"=w94:T14)  [unwired: 8 in]
          }
          event "Lichtgitter manuell ansteuern": Value Change {
            # "Hier können die Lichtgitter manuell und mit verschiedenen Befehlen angesteuert werden."
            n48 = event-data() -> ()  [unwired: 1 in, 6 out]
            n49 = call "Test_DL-EN1.vi"("Fehler in"=w104, "ID Messverstärker"="ID Messverstärker", "Befehl"="Befehl:", "Cluster in"=w103) -> ("Fehler out"=w102:errorcluster, "Lichtgitter Cluster out"=→"Ergebnisse:":T10, "Cluster out"=w101:T14)  [unwired: 4 in, 1 out]
          }
          event "Artikelnummer Offline": Value Change {
            # "Artikelnummer Offline ändern"
            n50 = event-data() -> ("NewVal"=w105:string)  [unwired: 1 in, 5 out]
            n51 = global write "Globale Variablen.vi" "Artikelnummer"(w105) -> ()
          }
          event "Offline.Start Gesamtablauf": Value Change {
            # "Offline- bzw. Manueller-Start. Wenn \"Start Offline\" betätigt wird und das Programm nicht im \"Online-Modus\" ist, werden alle Prüfungen, also Prüfung Oben, Vermessung Lichtgitter, Prüfung Unten\nautomatisch nacheinander ausgeführt."
            n52 = event-data() -> ("NewVal"=w111:bool)  [unwired: 1 in, 5 out]
            n53 = Bundle By Name(cluster=w109, "Einstellungen.Gesamtablauf gestartet"=w111) -> (w110:T14)
          }
          event "Offline.Teile-Datum": Value Change {
            # "Teile-Datums Ordner für Offline Teile ändern"
            n54 = event-data() -> ("NewVal"=w133:u16)  [unwired: 1 in, 5 out]
            n55 = Unbundle By Name(w128) -> ("Initialisierung.Grundpfad"=w125:path, "Artikeldaten.Artikelnummer"=w126:string)
            n56 = property on="Teile-Datum" class="Ring (strict)"() -> ("Strings []"=w130:string[])  [unwired: 2 in, 2 out]
            n57 = Build Path(base path=w125, name or relative path=path "Dateien") -> (appended path=w124:path)
            n58 = Index Array(array=w130, index=w133) -> (element=w120:string)
            n59 = Build Path(base path=w124, name or relative path=w126) -> (appended path=w123:path)
            n60 = Build Path(base path=w123, name or relative path=path "Bilder") -> (appended path=w121:path)
            n61 = Build Path(base path=w121, name or relative path=w120) -> (appended path=w119:path)
            n62 = Bundle By Name(cluster=w128, "Einstellungen.Ausgewähltes Offline-Teil"="0", "Einstellungen.Ausgewähltes Offline-Datum"=w120) -> (w129:T14)
            n63 = List Folder(path=w119, error in=w118) -> (folder names=w117:string[], error out=w114:errorcluster)  [unwired: 2 in, 2 out]
            n64 = Array Size(array=w117) -> (size(s)=w116:i32)
            n65 = Decrement(x=w116) -> (x-1=w115:i32)
            n66 = property on="Teile-Nummer" class="DigNum (strict)"("Value"=u32 0 ("Offline Teile-Nummer"), "Maximum"=w115) -> ()  [unwired: 2 in, 2 out]
          }
          event "Offline.Teile-Nummer": Value Change {
            # "Teile-Nummer für Offline-Prüfung ändern"
            n67 = event-data() -> ("NewVal"=w137:u32)  [unwired: 1 in, 5 out]
            n68 = Number To Decimal String(number=w137) -> (decimal integer string=w136:string)  [unwired: 1 in]
            n69 = Bundle By Name(cluster=w139, "Einstellungen.Ausgewähltes Offline-Teil"=w136) -> (w138:T14)
          }
          event "Offline.Kontaktnummer": Value Change {
            n70 = event-data() -> ("NewVal"=w144:u32)  [unwired: 1 in, 5 out]
            n71 = Bundle By Name(cluster=w145, "Artikeldaten.Aktueller Kontakt"=w144) -> (w142:T14)
          }
          event "SubVI öffnen": Value Change {
            # "SubVI öffnen"
            n72 = event-data() -> ()  [unwired: 1 in, 6 out]
            n73 = call "SubVI_oeffnen.vi"("error in"=w149, "Cluster in"=w150) -> ("error out"=w148:errorcluster, "Cluster out"=w147:T14)  [unwired: 8 in]
          }
          event "Cluster beobachten": Value Change {
            # "Öffnet ein VI, in dem das Cluster live angezeigt wird"
            n74 = event-data() -> ()  [unwired: 1 in, 6 out]
            n75 = Unbundle By Name(w156) -> ("Initialisierung.Online?"=w155:bool)
            n76 = Select(t=path "data/Cluster_beobachten.vi" ("Name oder relativer Pfad"), s=w155, f=path "SubVIs/Sonstige/Cluster_beobachten.vi" ("Name oder relativer Pfad")) -> (s? t:f=w152:path)
            n77 = call <vilib>:"Application Directory.vi"() -> ("Application Directory"=w165:path)
            n78 = Build Path(base path=w165, name or relative path=w152) -> (appended path=w151:path)
            n79 = Open VI Reference(vi path=w151) -> (vi reference=w164:refnum<vi>, error out=w162:errorcluster)  [unwired: 5 in]
            n80 = invoke class="VI" method="FP.Open"(reference=w164, error in=w162) -> (reference out=w163:refnum<vi>, error out=w161:errorcluster)  [unwired: 3 in, 3 out]
            n81 = Close Reference(reference=w163, error in (no error)=w161) -> (error out=w158:errorcluster)
            n82 = Merge Errors(w160, w158) -> (w159:errorcluster)
          }
          event "Zoom zurücksetzen": Value Change {
            w167 = cluster{"X":i32, "Y":i32} {"X"=-3, "Y"=-3} ("ZoomInteger:All Elements")
            w166 = cluster{"X":u32, "Y":u32} {"X"=2300, "Y"=2315} ("Image Center Position:All Elements")
            # "Zoom zurücksetzen"
            n83 = event-data() -> ()  [unwired: 1 in, 6 out]
            n84 = property on="Rohbild Referenzmarken" class="ImageControl"("Zoom to Fit Mode"=TRUE) -> ()  [unwired: 2 in, 2 out]
            n85 = property on="Rohbild ISO" class="ImageControl"("ZoomInteger"=w167, "Image Center Position"=w166) -> ()  [unwired: 2 in, 2 out]
            n86 = property on="Ermittlung Kontaktposition" class="ImageControl"("ZoomInteger"=w167, "Image Center Position"=w166) -> ()  [unwired: 2 in, 2 out]
            n87 = property on="Nachprüfung von Unten" class="ImageControl"("ZoomInteger"=cluster{"X":i32, "Y":i32} {"X"=-2, "Y"=-2} ("ZoomInteger:All Elements"), "Image Center Position"=cluster{"X":u32, "Y":u32} {"X"=1650, "Y"=950} ("Image Center Position:All Elements")) -> ()  [unwired: 2 in, 2 out]
          }
          event "Fehlercode:": Value Change {
            n88 = event-data() -> ()  [unwired: 1 in, 6 out]
            n89 = call "Fehlercode_suchen.vi"("Fehler in"=w179, "Fehlercode"="Fehlercode:", "Cluster in"=w178) -> ("Fehler out"=w177:errorcluster, "Fehlerbeschreibung"=→"Beschreibung:":string, "Cluster out"=w180:T14)  [unwired: 6 in]
          }
          event "ACK": Value Change {
            # "Löscht den Fehler in der Zustandsautomat-Schleife"
            n90 = event-data() -> ()  [unwired: 1 in, 6 out]
          }
          event Panel Close? {
            # "Programm wird mit schließen des Fensters beendet (haben wir bis jetzt bei noch keinem Automaten so gemacht, ist aber denke ich sinvoller als mit \"Programm beenden\"-Button)"
            n91 = event-data() -> ()  [unwired: 1 in, 4 out]
            n92 = global write "Globale Variablen.vi" "Programm beenden"(TRUE ("Programm beenden")) -> ()
            n93 = call "Dateien_updaten.vi"("Fehler in"=w192, "Cluster in"=w189) -> ("Fehler out"=w191:errorcluster, "Cluster out"=w190:T14)  [unwired: 8 in]
            n94 = Unbundle By Name(w190) -> ("Initialisierung.Kamera Oben"=w196:T15, "Initialisierung.Flüssiglinse"=w195:refnum<k5>, "Initialisierung.Kamera Unten"=w194:T15, "Initialisierung.Lichtgitter"=w193:refnum<k5>, "Initialisierung.Online?"=w185:bool)
            n95 = case shown="True" w185 {
              tunnel: w196 -> [_ w208]
              tunnel: w195 -> [_ w207]
              tunnel: w194 -> [_ w206]
              tunnel: w193 -> [_ w205]
              frame False {
              }
              frame True {
                n96 = call <vilib>:"IMAQdx Close Camera.vi"("Session In"=w208) -> ("error out"=w204:errorcluster)  [unwired: 10 in]
                n97 = TCP Close Connection(connection ID=w207) -> (error out=w203:errorcluster)  [unwired: 2 in, 1 out]
                n98 = call <vilib>:"IMAQdx Close Camera.vi"("Session In"=w206) -> ("error out"=w202:errorcluster)  [unwired: 10 in]
                n99 = TCP Close Connection(connection ID=w205) -> (error out=w201:errorcluster)  [unwired: 2 in, 1 out]
                n100 = Merge Errors(w204, w203, w202, w201) -> (→"Fehler Beenden":errorcluster)
              }
            }
            n101 = Not(x=w185) -> (.not. x?=w184:bool)
            n102 = flat-sequence {
              tunnel: w184 -> [w199]
              tunnel: [w199] -> w186
              frame #0 {
                n103 = Wait (ms)(milliseconds to wait=u32 200) -> ()  [unwired: 1 out]
              }
            }
            n104 = event-data("Discard?"=w186) -> ()  [unwired: 1 in, 1 out]
          }
        }
      }
      frame "Artikeldaten laden" {
        # "Wartezeit bis die globalen Variablen geladen sind"
        # "Bei Änderung der Artikelnummer werden hier alle Artikeldaten geladen"
        n105 = global read "Globale Variablen.vi" "Fertigungsauftrag"() -> (w211:string)
        n106 = global read "Globale Variablen.vi" "Artikelnummer"() -> (w212:string)
        n107 = Bundle By Name(cluster=T3 {"Artikelnummer"="", "Fertigungsauftrag"=""} ("Auftragsdaten"), "Artikelnummer"=w212, "Fertigungsauftrag"=w211) -> (→"Artikelnummer & Fertigungsauftrag":T3)
        n108 = Bundle By Name(cluster=w231, "Artikeldaten.Artikelnummer"=w212, "Artikeldaten.Fertigungsauftrag"=w211) -> (w224:T14)
        n109 = global write "Globale Variablen.vi" "Artikeldaten von SPS laden"(TRUE ("Artikeldaten laden")) -> ()
        n110 = flat-sequence {
          tunnel: w224 -> [w234]
          tunnel: [w234] -> w223
          frame #0 {
            n111 = Wait (ms)(milliseconds to wait=u32 1000) -> ()  [unwired: 1 out]
          }
        }
        n112 = call "Artikeldaten_laden.vi"("Fehler in"=w229, "Cluster in"=w223) -> ("Fehler out"=w230:errorcluster, "Anzahl Bilder out"=w225:i32, "Offline Teile-Datum out"=w227:string[], "Cluster out"=w221:T14)  [unwired: 6 in]
        n113 = Unbundle By Name(w221) -> ("Statistik.Statistiken"=w220:T6[])
        n114 = property on="Teile-Datum" class="Ring (strict)"("Strings []"=w227, "Value"=u16 0) -> ()  [unwired: 2 in, 2 out]
        n115 = property on="Kontaktnummer" class="DigNum (strict)"("Value"=u32 1) -> ()  [unwired: 2 in, 2 out]
        n116 = property on="Teile-Nummer" class="DigNum (strict)"("Value"=u32 0 ("Offline Teile-Nummer"), "Maximum"=w225) -> ()  [unwired: 2 in, 2 out]
        n117 = Index Array(array=w220, index #1=0 ("index"), index #2=1 ("index"), index #3=2 ("index")) -> (element #1=→"Statistik Anlage":T6, element #2=→"Statistik Artikel":T6, element #3=→"Statistik Auftrag":T6)
      }
      frame "Init Prüfung Oben" {
        w235 = T2 refnum ("Referenzbohrungen")
        # "Initialisierung der Oberen Prüfung"
        n118 = local write "Rohbild Referenzmarken"(w235) -> ()
        n119 = local write "Rohbild ISO"(w235) -> ()
        n120 = local write "Ermittlung Kontaktposition"(w235) -> ()
        n121 = invoke on="Messdaten" class="Clust (strict)" method="Reinit To Default"() -> ()  [unwired: 3 in, 3 out]
        n122 = call "Init_Pruefung_Oben.vi"("Fehler in"=w240, "Cluster in"=w241) -> ("Fehler out"=w238:errorcluster, "Cluster out"=w239:T14)  [unwired: 8 in]
        n123 = call "Ergebnis_an_SPS.vi"("error in"=w238, "Cluster in"=w239) -> ("error out"=w237:errorcluster, "Cluster out"=w236:T14)  [unwired: 8 in]
      }
      frame "Bildaufnahme Oben" {
        # "Bildaufnahme für die Obere Prüfung (Referenzbohrungen, ISO und Nachkontrolle des vorher montierten Kontakts)"
        n124 = call "Bildaufnahme_Oben.vi"("Fehler in"=w250, "Cluster in"=w251) -> ("Fehler out"=w245:errorcluster, "Cluster out"=w248:T14)  [unwired: 8 in]
        n125 = call "Lichtgitter_Referenzen_aufnehmen.vi"("Fehler in"=w250, "Cluster in"=w251) -> ("Fehler out"=w243:errorcluster, "Cluster out"=w249:T14)  [unwired: 8 in]
        n126 = Unbundle By Name(w249) -> ("Werte Lichtgitter"=w246:T21)
        n127 = Bundle By Name(cluster=w248, "Werte Lichtgitter"=w246) -> (w247:T14)
        n128 = Merge Errors(w245, w243) -> (w244:errorcluster)
      }
      frame "Auswertung Oben" {
        # "Auswertung der Oberen Prüfung"
        n129 = call "Verarbeitung_Oben.vi"("Fehler in"=w284, "Größe Kontaktsuchfeld"="Größe Kontaktsuchfeld", "Cluster in"=w259) -> ("Fehler out"=w261:errorcluster, "Cluster out"=w262:T14)  [unwired: 7 in]
        n130 = Unbundle By Name(w262) -> ("Timer.Timer Start Position"=w265:u32, "Initialisierung.Bilder Oben"=w289:T2[], "Werte Kamera Oben.Position Kontakt umgerechnet"=w257:cluster{"x":dbl, "y":dbl}, "Werte Kamera Oben.Winkel Kontakt"=w256:dbl, "Werte Kamera Oben.Durchmesser Loch"=w253:dbl, "Artikeldaten.Aktueller Kontakt"=w282:i16, "Initialisierung.Online?"=w277:bool, "Einstellungen.Bildspeicherung Offline"=w271:bool, "Fehler.Kontakt nicht gefunden"=w269:bool, "Einstellungen.Gesamtablauf gestartet"=w270:bool)
        n131 = call "Ergebnis_an_SPS.vi"("error in"=w261, "Cluster in"=w262) -> ("error out"=w260:errorcluster, "Cluster out"=w258:T14)  [unwired: 8 in]
        n132 = Or(x=w277, y=w271) -> (x .or. y?=w276:bool)
        n133 = flat-sequence {
          tunnel: w265 -> [w291]
          tunnel: [w290] -> w274
          tunnel: w260 -> [_]
          frame #0 {
            n134 = Tick Count (ms)() -> (millisecond timer value=w292:u32)
            n135 = Subtract(x=w292, y=w291) -> (x-y=w290:u32)
          }
        }
        n136 = local read "Messdaten"() -> (w254:T4)
        n137 = Bundle By Name(cluster=w254, "Position Kontakt"=w257, "Winkel Kontakt"=w256, "Durchmesser Loch"=w253) -> (→"Messdaten":T4)
        n138 = Index Array(array=w289, index #1=0 ("index"), index #2=1 ("index"), index #3=2 ("index")) -> (element #1=→"Rohbild Referenzmarken":T2, element #2=→"Rohbild ISO":T2, element #3=→"Ermittlung Kontaktposition":T2)
        n139 = Equal?(x=i16 1 ("y"), y=w282) -> (x = y?=w279:bool)
        n140 = And(x=w279, y=w276) -> (x .and. y?=w278:bool)
        n141 = Select(t=Zustand."Init Vermessung Lichtgitter", s=w270, f=Zustand."Warten auf Event" ("t")) -> (s? t:f=w268:T11)
        n142 = Select(t=Zustand."Update Statistik", s=w269, f=w268) -> (s? t:f=w266:T11)
        n143 = Select(t=Zustand."Bilder Oben speichern", s=w278, f=w266) -> (s? t:f=w283:T11)
        "Zeit Position ermitteln (ms)" <- w274
      }
      frame "Bilder Oben speichern" {
        n144 = call "Bilder_Oben_speichern.vi"("Fehler in"=w302, "Cluster in"=w303) -> ("Fehler out"=w301:errorcluster, "Cluster out"=w299:T14)  [unwired: 8 in]
        n145 = Unbundle By Name(w299) -> ("Fehler.Kontakt nicht gefunden"=w296:bool, "Einstellungen.Gesamtablauf gestartet"=w300:bool)
        n146 = Select(t=Zustand."Init Vermessung Lichtgitter" ("State"), s=w300, f=Zustand."Warten auf Event" ("State")) -> (s? t:f=w295:T11)
        n147 = Select(t=Zustand."Update Statistik", s=w296, f=w295) -> (s? t:f=w294:T11)
      }
      frame "Init Vermessung Lichtgitter" {
        w304 = FALSE ("Fehler.Kontakt zu klein")
        # "Initialisierung der Vermessung im Lichtgitter"
        n148 = Tick Count (ms)() -> (millisecond timer value=w307:u32)
        n149 = Bundle By Name(cluster=w306, "Timer.Timer Start Lichtgitter"=w307, "Fehler.Referenzen nicht in Lichtgitter"=w304, "Fehler.Kontakt zu groß"=w304, "Fehler.Kontakt zu klein"=w304) -> (w310:T14)
        n150 = call "Ergebnis_an_SPS.vi"("error in"=w305, "Cluster in"=w310) -> ("error out"=w309:errorcluster, "Cluster out"=w308:T14)  [unwired: 8 in]
      }
      frame "Messwertaufnahme Lichtgitter" {
        # "Messwertaufnahme der Lichtgitter"
        n151 = call "Aufnahme_Lichtgitter.vi"("Fehler in"=w314, "Cluster in"=w315) -> ("Fehler out"=w312:errorcluster, "Cluster out"=w313:T14)  [unwired: 8 in]
      }
      frame "Auswertung Lichtgitter" {
        # "Auswertung der Lichtgitter-Messwerte"
        n152 = call "Auswertung_Lichtgitter.vi"("Fehler in"=w334, "Cluster in"=w335) -> ("Fehler out"=w329:errorcluster, "Durchmesser Kontakt (mm)"=w317:dbl, "Cluster out"=w328:T14)  [unwired: 7 in]
        n153 = Unbundle By Name(w328) -> ("Timer.Timer Start Lichtgitter"=w323:u32, "Initialisierung.Bilder Oben"=w320:T2[], "Einstellungen.Gesamtablauf gestartet"=w333:bool, "Werte Lichtgitter.Offset"=w319:cluster{"x":dbl, "y":dbl})
        n154 = call "Ergebnis_an_SPS.vi"("error in"=w329, "Cluster in"=w328) -> ("error out"=w322:errorcluster, "Cluster out"=w327:T14)  [unwired: 8 in]
        n155 = flat-sequence {
          tunnel: w323 -> [w337]
          tunnel: [w336] -> w326
          tunnel: w322 -> [_]
          frame #0 {
            n156 = Tick Count (ms)() -> (millisecond timer value=w338:u32)
            n157 = Subtract(x=w338, y=w337) -> (x-y=w336:u32)
          }
        }
        n158 = Index Array(array=w320, index=2) -> (element=w331:T2)
        n159 = local read "Messdaten"() -> (w321:T4)
        n160 = Bundle By Name(cluster=w321, "Offset"=w319, "Durchmesser Kontakt"=w317) -> (w318:T4)
        n161 = local write "Ermittlung Kontaktposition"(w331) -> ()
        n162 = local write "Messdaten"(w318) -> ()
        n163 = Select(t=Zustand."Init Prüfung Unten" ("State"), s=w333, f=Zustand."Warten auf Event" ("State")) -> (s? t:f=w332:T11)
        "Zeit Lichtgitter (ms)" <- w326
      }
      frame "Init Prüfung Unten" {
        # "Initialisierung der Unteren Prüfung"
        n164 = local write "Nachprüfung von Unten"(T2 refnum ("Bild unten")) -> ()
        n165 = Tick Count (ms)() -> (millisecond timer value=w340:u32)
        n166 = Bundle By Name(cluster=w345, "Werte Kamera Unten"=cluster{"Prüfung Unten n. i. O.":bool} {"Prüfung Unten n. i. O."=FALSE}, "Timer.Timer Start Kamera Unten"=w340) -> (w344:T14)
        n167 = call "Ergebnis_an_SPS.vi"("error in"=w341, "Cluster in"=w344) -> ("error out"=w342:errorcluster, "Cluster out"=w343:T14)  [unwired: 8 in]
      }
      frame "Bildaufnahme Unten" {
        # "Bildaufnahme der Unteren Prüfung (Nur ein Bild)"
        n168 = call "Bildaufnahme_Unten.vi"("Fehler in"=w353, "Cluster in"=w355) -> ("Fehler out"=w352:errorcluster, "Bild existiert?"=w349:bool, "Cluster out"=w354:T14)  [unwired: 7 in]
        n169 = Select(t=Zustand."Auswertung Unten" ("State"), s=w349, f=Zustand."Warten auf Event") -> (s? t:f=w351:T11)
      }
      frame "Auswertung Unten" {
        # "Auswertung der Unteren Prüfung"
        n170 = call "Verarbeitung_Unten.vi"("Fehler in"=w370, "Cluster in"=w371) -> ("Fehler out"=w368:errorcluster, "Cluster out"=w367:T14)  [unwired: 8 in]
        n171 = Unbundle By Name(w367) -> ("Timer.Timer Start Kamera Unten"=w357:u32, "Initialisierung.Bild Unten"=→"Nachprüfung von Unten":T2, "Initialisierung.Online?"=w365:bool, "Einstellungen.Bildspeicherung Offline"=w361:bool)
        n172 = call "Ergebnis_an_SPS.vi"("error in"=w368, "Cluster in"=w367) -> ("error out"=w356:errorcluster, "Cluster out"=w359:T14)  [unwired: 8 in]
        n173 = flat-sequence {
          tunnel: w357 -> [w374]
          tunnel: [w373] -> w362
          tunnel: w356 -> [_]
          frame #0 {
            n174 = Tick Count (ms)() -> (millisecond timer value=w375:u32)
            n175 = Subtract(x=w375, y=w374) -> (x-y=w373:u32)
          }
        }
        n176 = Bundle By Name(cluster=w359, "Einstellungen.Gesamtablauf gestartet"=FALSE) -> (w358:T14)
        n177 = Or(x=w365, y=w361) -> (x .or. y?=w364:bool)
        n178 = Select(t=Zustand."Bild Unten speichern" ("State"), s=w364, f=Zustand."Update Statistik" ("State")) -> (s? t:f=w372:T11)
        "Zeit Kamera Unten (ms)" <- w362
      }
      frame "Bild Unten speichern" {
        # "Speichern der Bilder der Nachkontrollen (Werden nach vollständigem Bestücken des ISOs oder wenn eine der beiden Nachkontrollen schlecht ist gespeichert (oder wenn die Kontaktnummer zurückgesetzt wird))"
        n179 = call "Bilder_Unten_speichern.vi"("Fehler in"=w378, "Cluster in"=w379) -> ("Fehler out"=w377:errorcluster, "Cluster out"=w376:T14)  [unwired: 8 in]
      }
      frame "Update Statistik" {
        n180 = call "Update_Statistik.vi"("error in"=w391, "Cluster in"=w389) -> ("error out"=w390:errorcluster, "Cluster out"=w388:T14)  [unwired: 8 in]
        n181 = Unbundle By Name(w388) -> ("Statistik.Statistiken"=w381:T6[])
        n182 = Index Array(array=w381, index #1=0 ("index"), index #2=1 ("index"), index #3=2 ("index")) -> (element #1=w387:T6, element #2=w385:T6, element #3=w386:T6)
        n183 = local write "Statistik Artikel"(w385) -> ()
        n184 = local write "Statistik Auftrag"(w386) -> ()
        n185 = local write "Statistik Anlage"(w387) -> ()
      }
      frame "Fehler quittieren" {
        n186 = Bundle By Name(cluster=w396, "Fehler"=T20 {"Referenzen nicht gefunden"=FALSE, "Kontakt nicht gefunden"=FALSE, "Kontakt nicht in Lichtgitter"=FALSE, "Kontakt zu groß"=FALSE, "Kontakt zu klein"=FALSE}) -> (w395:T14)
        n187 = call "Quittieren_SPS.vi"("error in"=errorcluster {"status"=FALSE, "code"=0, "source"=""} ("Fehler out"), "Cluster in"=w395) -> ("error out"=w397:errorcluster, "Cluster out"=w398:T14)  [unwired: 8 in]
      }
    }
    n188 = call "Cluster_beobachten.vi"("error in"=w28, "Cluster in"=w34) -> ("error out"=w27:errorcluster, "Cluster out"=w31:T14)  [unwired: 8 in]
    "Zustand" <- w29
    "Fehler Main" <- w36
  }
  n189 = while {
    shift-right: [w429] -> _
    shift-left: errorcluster {"status"=FALSE, "code"=0, "source"=""} ("error out") -> [w419]
    shift-right: [w417] -> _
    shift-left: w6 -> [w418]
    tunnel: w9 -> [w408]
    shift-right: [w403] -> _
    shift-left: T7 {"Artikelnummer"="", "Fertigungsauftrag"="", "Start Position ermitteln"=FALSE, "Start Kontaktvermessung Lichtgitter"=FALSE, "Start Nachkontrolle"=FALSE, "ACK SPS"=FALSE} ("SPS IN") -> [w406]
    stop <- w430 stop-if-true
    # "Hier ist alles, was nicht in den Zustandsautomaten passt. Also alles was kontinuierlich laufen soll"
    n190 = Wait (ms)(milliseconds to wait=u32 10 ("Zu wartende ms")) -> ()  [unwired: 1 out]
    n191 = local read "Fehler Kamera Unten"() -> (w411:errorcluster)
    n192 = local read "Fehler init allgemein"() -> (w414:errorcluster)
    n193 = local read "Fehler Kamera Oben"() -> (w413:errorcluster)
    n194 = global read "Globale Variablen.vi" "Fehlermeldung SPS"() -> (w409:errorcluster)
    n195 = local read "Fehler Flüssiglinse"() -> (w412:errorcluster)
    n196 = local read "Fehler Lichtgitter"() -> (w410:errorcluster)
    n197 = local read "Fehler Main"() -> (w415:errorcluster)
    n198 = property on="Registerkarte" class="TabCtl (strict)"() -> ("Pages"=w421:refnum<vi>[])  [unwired: 2 in, 2 out]
    n199 = Index Array(array=w421, index=4) -> (element=w425:refnum<vi>)
    n200 = local write "Fehler SPS"(w409) -> ()
    n201 = Compound Arithmetic op=OR(w419, w415, w414, w413, w412, w411, w410, w409) -> (w420:bool)
    n202 = Select(t=u32 16711680, s=w420, f=u32 12369084) -> (s? t:f=w426:u32)
    n203 = property class="Page"(reference=w425, "FG Color"=w426) -> ()  [unwired: 1 in, 2 out]
    n204 = call "SPS-Variablen_nach_Cluster.vi"("Fehler in"=w419, "Cluster in"=w418) -> ("Fehler out"=w416:errorcluster, "SPS OUT"=→"SPS OUT":T8, "SPS IN"=w407:T7, "Cluster out"=w417:T14)  [unwired: 6 in]
    "SPS IN" <- w407
    n205 = call "Flankenauswertung_SPS.vi"("SPS IN"=w407, "Schieberegister in"=w406) -> ("Event out"=w404:T11, "Positive Flanke"=w405:bool, "Schieberegister out"=w403:T7)  [unwired: 7 in]
    n206 = global read "Globale Variablen.vi" "Programm beenden"() -> (w430:bool)
    n207 = local read "ACK"() -> (w401:bool)
    n208 = case shown="True" w405 {
      tunnel: w408 -> [_ w432]
      tunnel: w404 -> [_ w431]
      frame False {
      }
      frame True {
        n209 = Generate User Event(user event=w432, event data cluster=w431) -> ()  [unwired: 2 in, 2 out]
      }
    }
    n210 = Select(t=errorcluster {"status"=FALSE, "code"=0, "source"=""}, s=w401, f=w416) -> (s? t:f=w429:errorcluster)
    n211 = local write "ACK"(FALSE ("ACK")) -> ()
    "Fehler Nebenschleife" <- w419
  }
